vi "Q14070-Z040轴向间隙测试台.vi"() -> ()   [LabVIEW 2013]
uses:
  <vilib>/Utility/file.llb/Write To Spreadsheet File (DBL).vi
  PCI8622_32.dll
panel:
  in  "确定按钮 3":bool
  in  "确定按钮 2":bool
  in  "确定按钮":bool
  in  "密码":string
  out "生产":bool
  out "source":string caption="源"
  out "code":i32 caption="代码"
  out "阻挡 2":bool
  out "error out 5":errorcluster
  out "型号数量":dbl
  in  "循环次数":u16
  out "旋转左极限位(mm)":dbl=-40.0
  out "旋转右极限位(mm)":dbl=60.0
  out "输入轴快进位置(mm)":dbl=-40.0
  out "输入轴初始位置(mm)":dbl=60.0
  out "输入轴最终位置（mm)":dbl format="%#.3f"
  out "左右基准":dbl=-40.0
  in  "进给速度":dbl=10.0
  in  "旋转速度":dbl=10.0
  out "DeviceHandle":u32
  out "输入轴电机慢进位置3":dbl format="%#.3f"
  out "输入轴电机慢进位置2":dbl format="%#.3f"
  out "旋转轴伺服位置":dbl=10000.0 format="%#.2f"
  out "复位按钮":bool=TRUE
  out "报警工步号":dbl
  out "报警信息":string
  out "输入轴伺服位置":dbl=10000.0 format="%#.1f"
  out "力矩（nm)":dbl format="%#.2f"
  out "位移(mm)":dbl format="%#.3f"
  in  "员工权限":bool=TRUE
  out "测试操作状态":string
  in  "测试 工步号":dbl
  out "通讯状态":bool
  in  "停止":bool
  out "流水线操作状态":string
  in  "流水线工步号":dbl
  in  "联线按钮":bool
  in  "选项卡控件 2":enum32{"间隙曲线", "手动", "传感器校验", "参数查询"}(tab)
  out "10Nm间隙值(mm)":dbl format="%#.3f"
  out "-10Nm间隙值(mm)":dbl format="%#.3f"
  out "检测扭矩(NM)":dbl format="%#.1f"
  out "轴向间隙值(mm)":dbl format="%#.3f"
  out "上序合格":bool
  out "上序不合格":bool
  out "本序合格":bool
  out "间隙合格标准值(mm)":dbl=0.2 format="%#.3f"
  out "换向扭矩(NM)":dbl format="%#.1f"
  out "XY图":cluster{dbl[], dbl[]}[](graph)
  out "本序已做":bool
  in  "旋转伺服使能":bool
  in  "输入轴使能":bool
  out "放行":bool
  in  "阻挡":bool
  in  "扳手无效":bool
  out "流水线气缸下限":bool
  out "流水线气缸上限":bool
  out "下工位检测":bool
  out "本工位检测":bool
  out "上工位检测":bool
  in  "M顶升气缸上升":bool
  in  "M顶升气缸下降":bool
  in  "M本阻挡器":bool
  in  "M上阻挡器":bool
  in  "电机回零":bool
  in  "电机下降":bool
  in  "电机上升":bool
  in  "左旋":bool
  in  "右旋":bool
  in  "扭矩传感器零点偏移":dbl format="%#.2f"
  in  "扭矩传感器比例偏移":dbl=1.0 format="%#.2f"
  in  "位移传感器零点偏移":dbl format="%#.2f"
  in  "位移传感器比例偏移":dbl=1.0 format="%#.2f"
  in  "传感器参数保存":bool
  in  "参数保存":bool
  in  "参数查询":bool
  in  "参数列表":string[][](table)
  out "员工ID":string
  out "员工姓名":string
  in  "型号选择":u16(ring) items=["J728", "J706", "J709"]
  in  "参数加载":bool
  out "产品ID":string
  out "轴向间隙比例系数":dbl=1.0 format="%#_2f"
  out "error out 2":errorcluster
  out "输入轴电机快进速度":dbl format="%#.1f"
  out "输入轴电机慢进速度":dbl format="%#.3f"
  out "旋转电机速度":dbl=5.0 format="%#.3f"
  out "ADODB._Connection Out":refnum<k7>
  out "error out 3":errorcluster
  out "error out":errorcluster
  out "急停按钮":bool=TRUE
  out "芯片ID":string
  out "旋转轴AxisHandle OUT":u32
  out "FGCS":string="0"
  out "RFID读取完成":bool
  out "RFID读取触发":bool
  out "Z040 RFID":string="A001"
  out "KSJJ":string
  out "ReturnValue 3":u32
  out "ReturnValue":u32
  out "输入轴AxisHandle OUT":u32
  out "产品选型":dbl
  # "齿轮轴轴向间隙测试台"
  # "Q14070机械转向器装配线"
  # "Copying (C) 2015 湖北唯思凌科装备制造有限公司 版权所有"
  # "≤"
  # "传感器校验区"
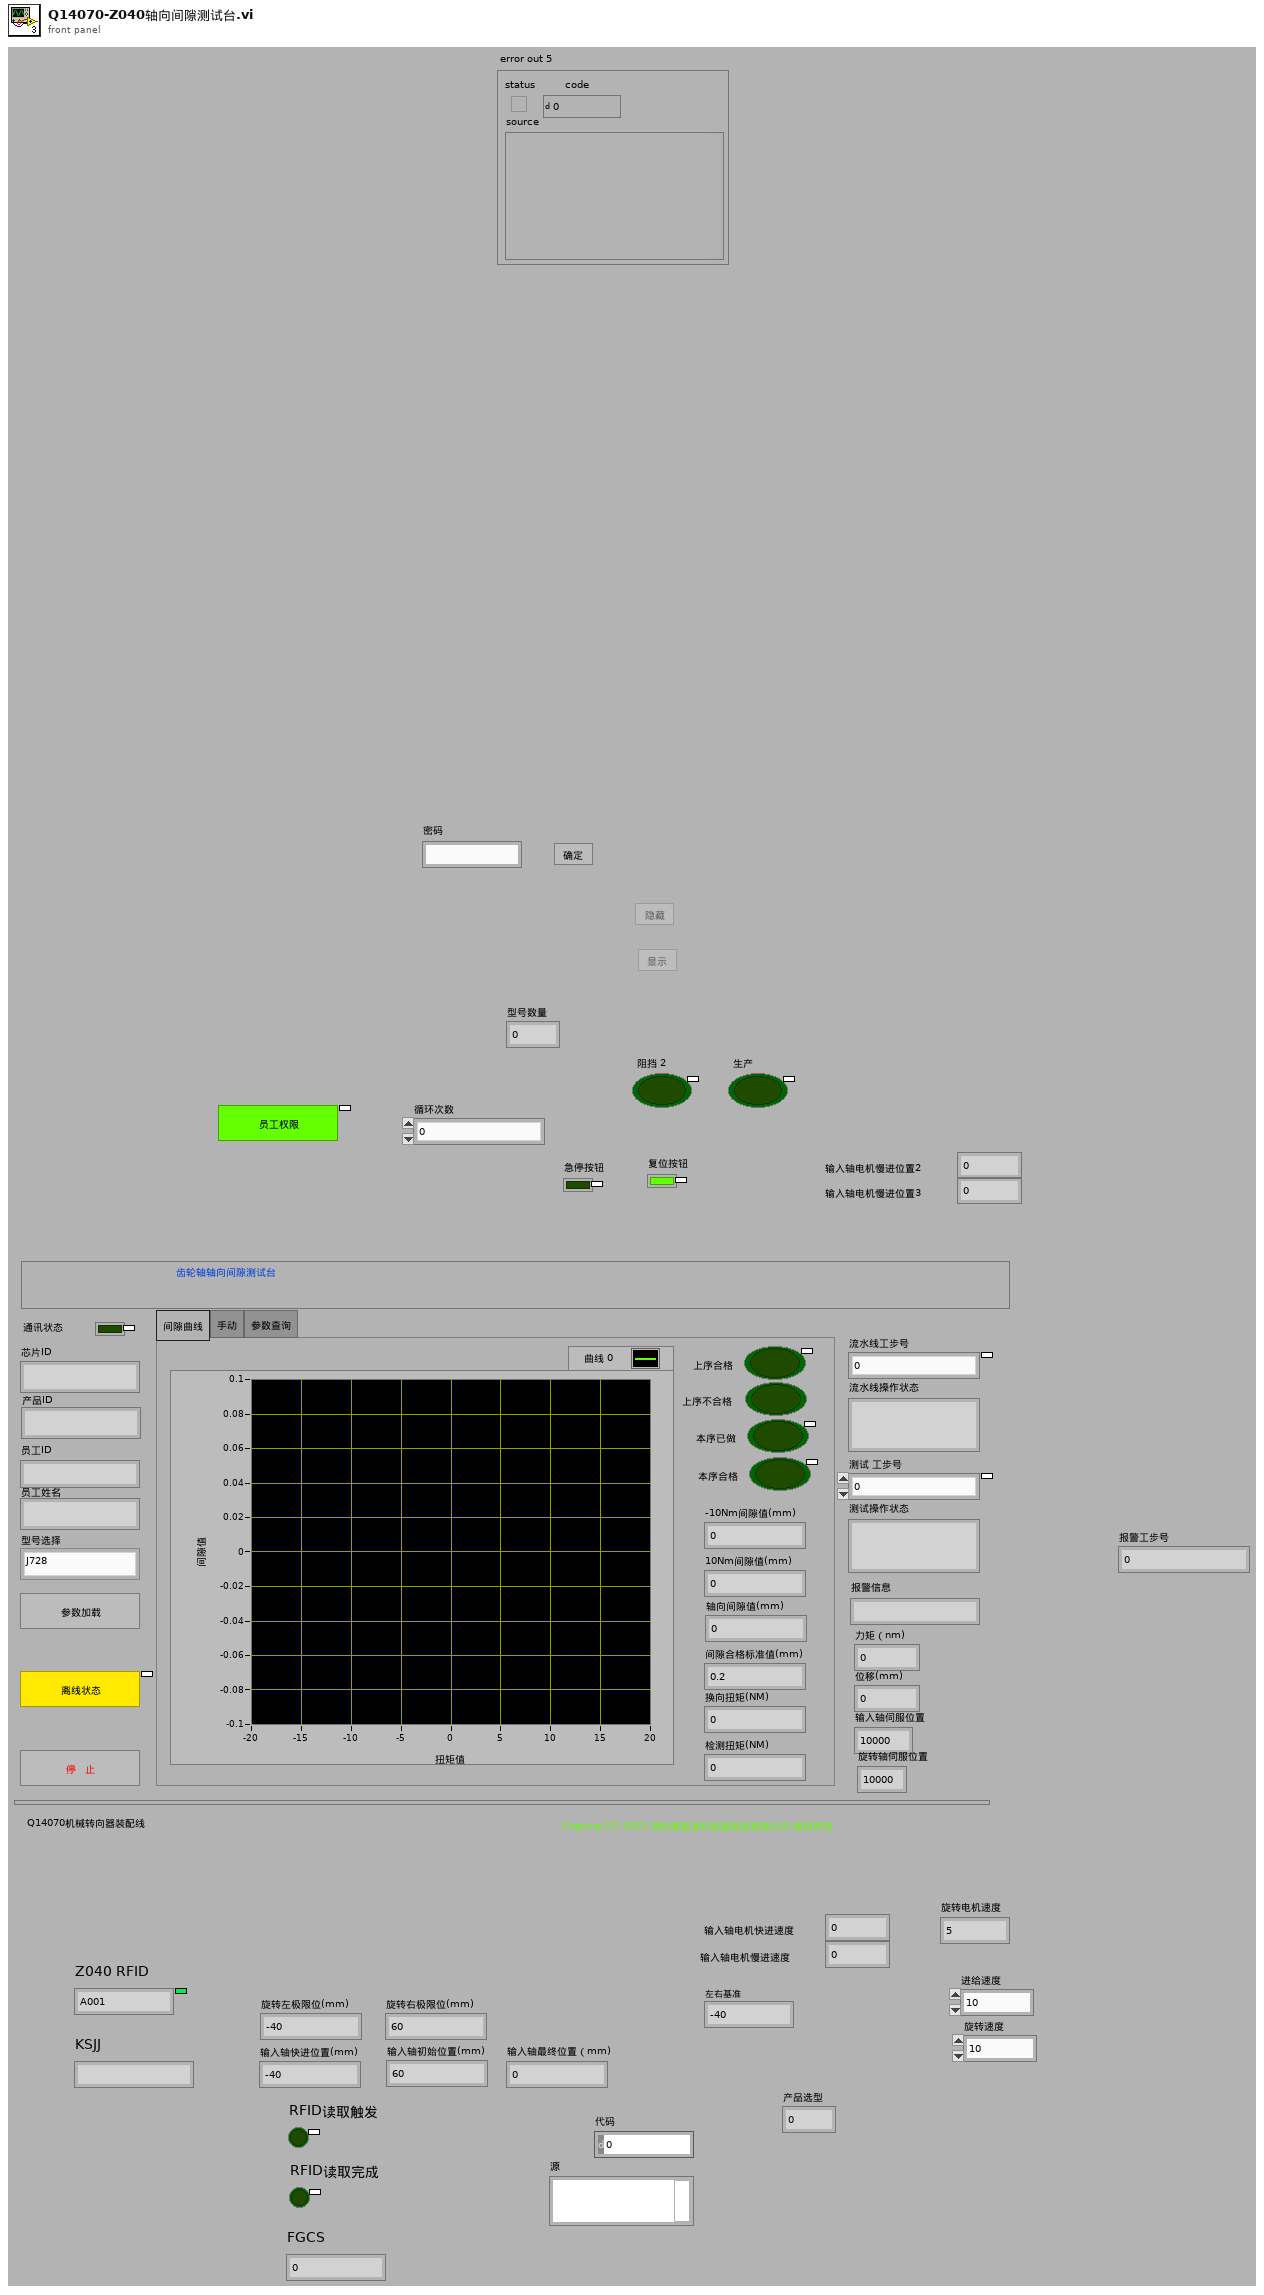
[diagram p1: front panel]
types:
  T1 = typedef "imagedata.ctl" = cluster{"image type":i32, "image depth":i32, "image":u8[], "mask":u8[], "colors":u32[], "Rectangle":cluster{"left":i16, "top":i16, "right":i16, "bottom":i16}}
  T2 = enum8{"Enabled", "Disabled", "Disabled and Grayed Out"}
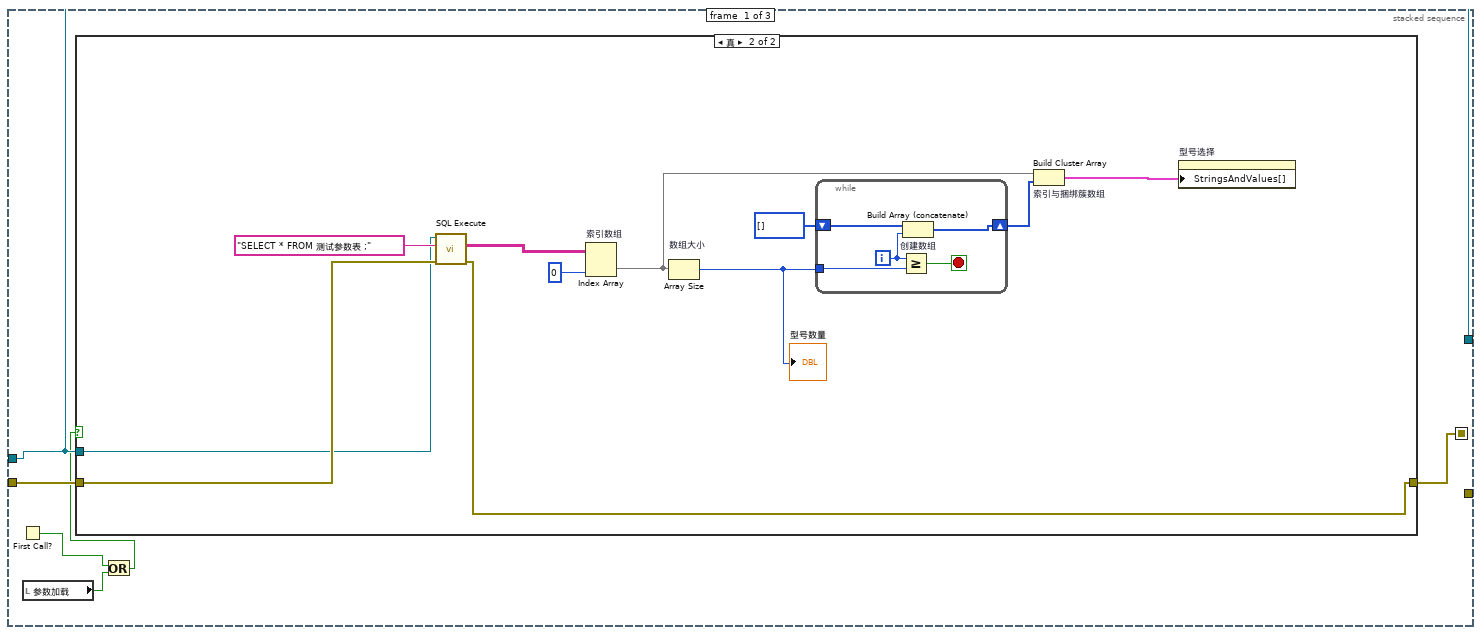
[diagram p3: hidden frame]
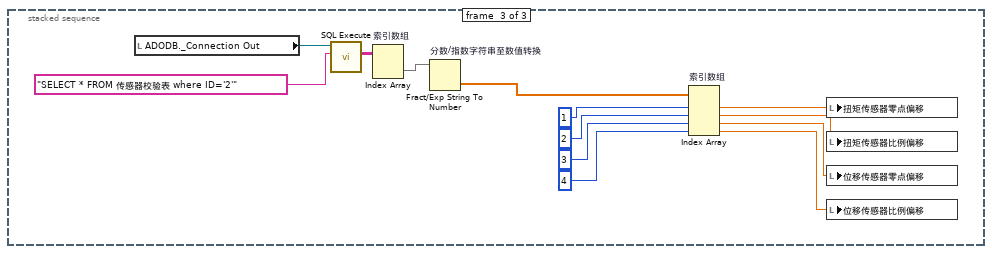
[diagram p5: hidden frame]
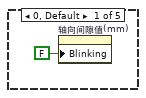
[diagram p6: hidden frame]
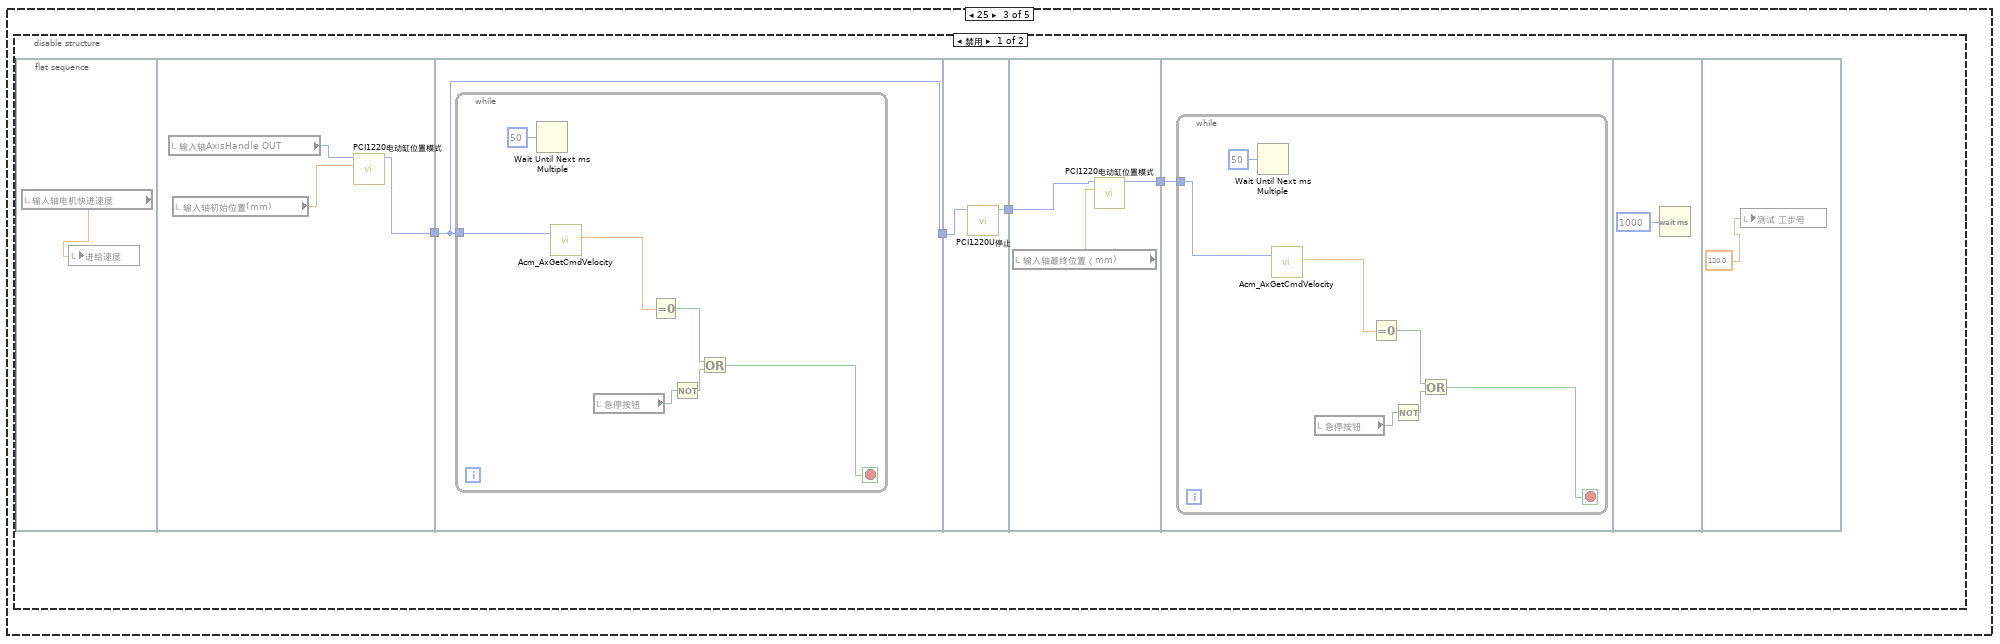
[diagram p8: hidden frame]
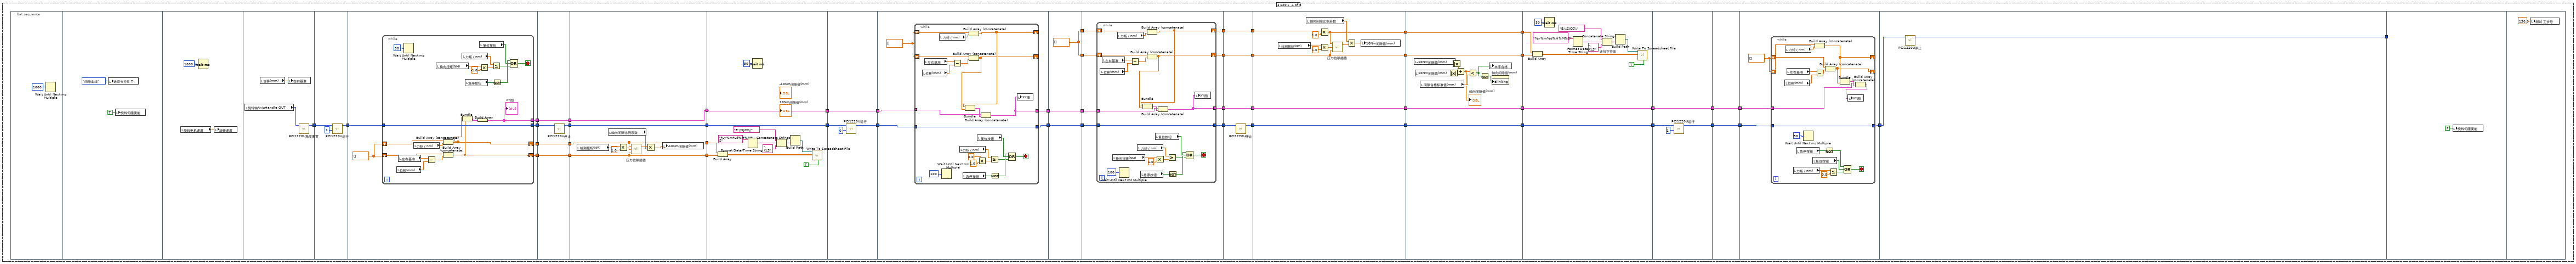
[diagram p10: hidden frame]
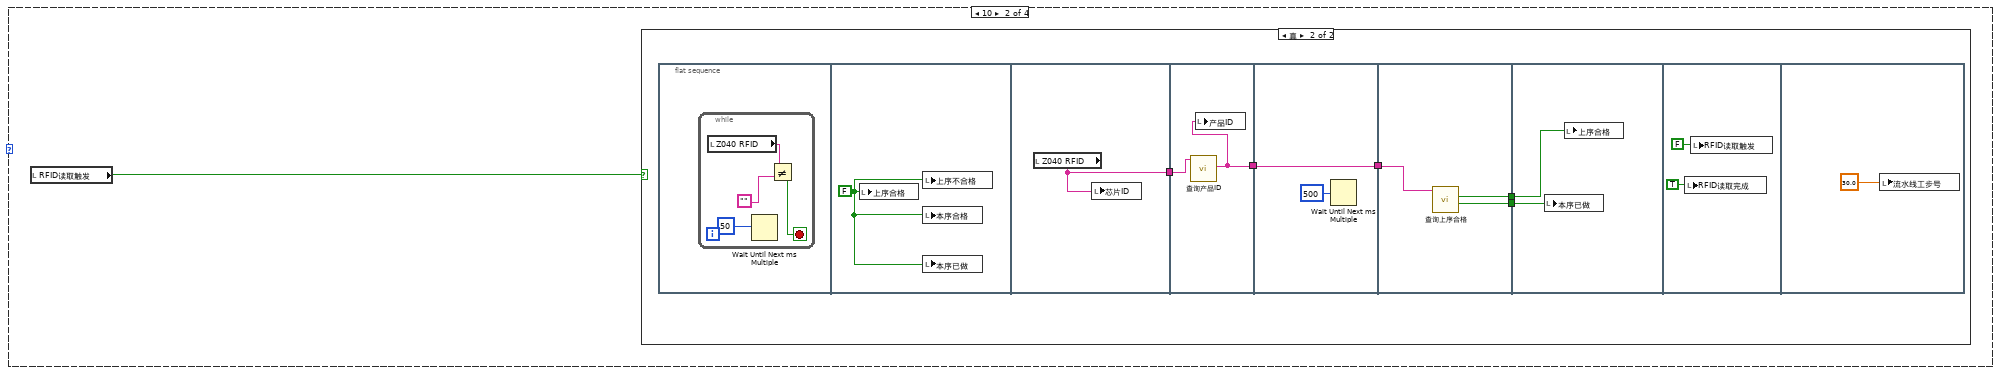
[diagram p12: hidden frame]
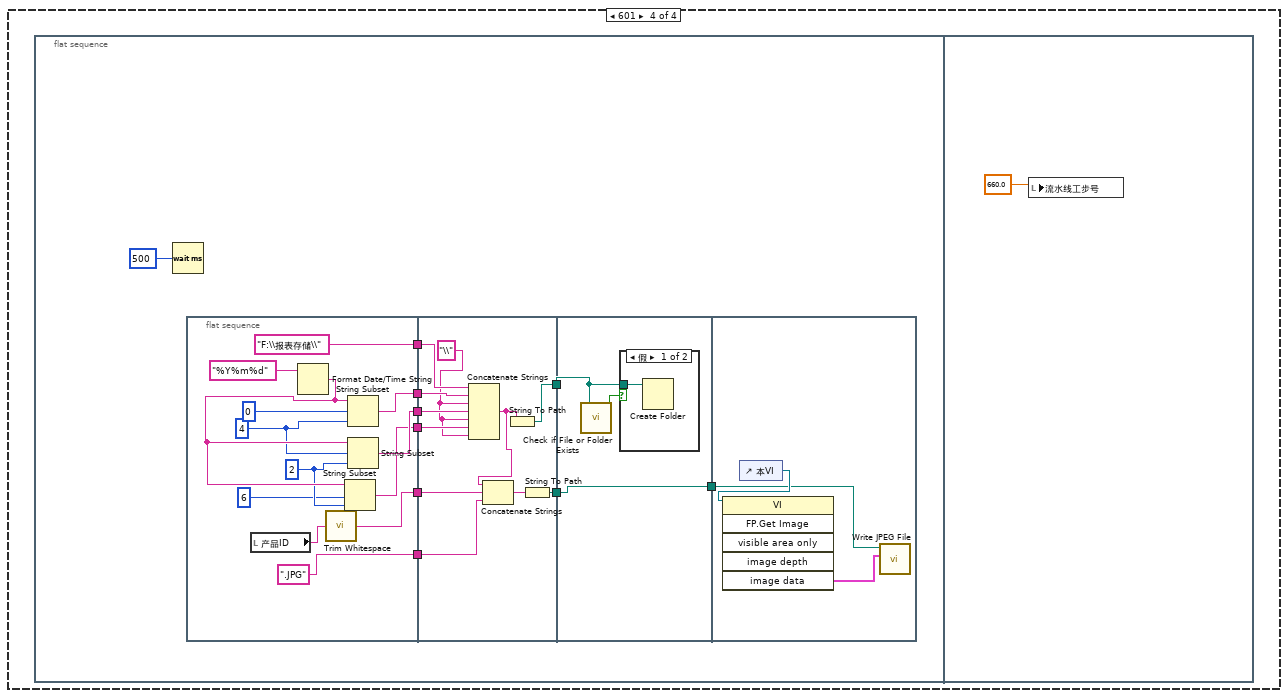
[diagram p15: hidden frame]
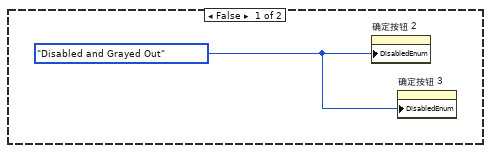
[diagram p17: hidden frame]
diagram:
  n1 = while {
    stop <- w10 stop-if-true
    n2 = local read "测试 工步号"() -> (w12:dbl)
    n3 = case shown="140" w12 {
      frame 0, Default {
        n4 = property on="轴向间隙值(mm)" class="DigNum (严格)"("Blinking"=FALSE ("闪烁")) -> ()  [unwired: 2 in, 2 out]
      }
      frame 20 {
        n5 = flat-sequence {
          tunnel: [w43] -> w14
          tunnel: w14 -> [w45]
          tunnel: [w45] -> w33
          tunnel: w33 -> [w47]
          tunnel: [w46] -> w35
          tunnel: w35 -> [w62]
          tunnel: [w64] -> w25
          tunnel: w25 -> [w67]
          tunnel: [w67] -> w24
          tunnel: w24 -> [w70]
          tunnel: [w70] -> w23
          tunnel: [w74] -> w30
          tunnel: w23 -> [w73]
          tunnel: [w71] -> w27
          tunnel: [w77] -> w32
          tunnel: w30 -> [w77]
          tunnel: [w78] -> w29
          tunnel: w27 -> [w78]
          tunnel: w32 -> [w81]
          tunnel: [w81] -> w31
          tunnel: w29 -> [w79]
          tunnel: [w79] -> w28
          tunnel: w31 -> [w85]
          tunnel: [w84] -> w34
          tunnel: w28 -> [w83]
          tunnel: [w82] -> w26
          tunnel: w34 -> [w104]
          tunnel: w26 -> [w101]
          tunnel: [w100] -> w22
          tunnel: w22 -> [w106]
          tunnel: [w106] -> w21
          tunnel: w21 -> [w107]
          tunnel: [w107] -> w20
          tunnel: w20 -> [w110]
          tunnel: [w110] -> w19
          tunnel: w19 -> [w112]
          tunnel: [w111] -> w15
          tunnel: w15 -> [w126]
          tunnel: [w125] -> w18
          tunnel: w18 -> [w128]
          tunnel: [w127] -> w17
          tunnel: w17 -> [w131]
          tunnel: [w131] -> w16
          tunnel: w16 -> [w132]
          frame #0 {
            w39 = 0.0
            n6 = local read "输入轴电机快进速度"() -> (w40:dbl)
            n7 = property on="轴向间隙值(mm)" class="DigNum (严格)"("Blinking"=FALSE ("闪烁")) -> ()  [unwired: 2 in, 2 out]
            n8 = Format Date/Time String(time format string (%c)="%Y%m%d%H%M" ("时间格式字符串(%c)")) -> (date/time string=w36:string)  [unwired: 2 in]
            n9 = local write "-10Nm间隙值(mm)"(w39) -> ()
            n10 = local write "10Nm间隙值(mm)"(w39) -> ()
            n11 = local write "轴向间隙值(mm)"(w39) -> ()
            n12 = local write "进给速度"(w40) -> ()
            n13 = local write "KSJJ"(w36) -> ()
          }
          frame #1 {
            n14 = local read "输入轴AxisHandle OUT"() -> (w41:u32)
            n15 = local read "输入轴快进位置(mm)"() -> (w42:dbl)
            n16 = call "PCI1220电动缸位置模式 .vi"("Distance"=w42, "AxisHandle IN"=w41) -> ("AxisHandle OUT"=w43:u32)  [unwired: 8 in, 1 out]
          }
          frame #2 {
            n17 = Wait (ms)(milliseconds to wait=u32 100 ("等待时间（毫秒）")) -> ()  [unwired: 1 out]
          }
          frame #3 {
            n18 = while {
              tunnel: w47 -> [w58]
              tunnel: [w59] -> w46
              stop <- w49 stop-if-true
              n19 = local read "力矩（nm)"() -> (w56:dbl)
              n20 = Wait Until Next ms Multiple(millisecond multiple=u32 50 ("毫秒倍数")) -> ()  [unwired: 1 out]
              n21 = Absolute Value(x=w56) -> (abs(x)=w55:dbl)
              n22 = call <userlib>:"Acm_AxGetCmdVelocity.vi"("AxisHandle"=w58) -> ("Velocity"=w60:dbl, "AxisHandle"=w59:u32)  [unwired: 1 in, 2 out]
              n23 = local read "急停按钮"() -> (w52:bool)
              n24 = Equal To 0?(x=w60) -> (x = 0?=w57:bool)
              n25 = local read "复位按钮"() -> (w48:bool)
              n26 = Greater Or Equal?(x=w55, y=15) -> (x >= y?=w53:bool)
              n27 = Or(x=w57, y=w53) -> (x .or. y?=w51:bool)
              n28 = Not(x=w52) -> (.not. x?=w50:bool)
              n29 = Compound Arithmetic op=OR(w48, w51, w50) -> (w49:bool)
            }
          }
          frame #4 {
            n30 = call "PCI1220U停止.vi"("AxisHandle IN"=w62) -> ()  [unwired: 9 in, 2 out]
          }
          frame #5 {
            n31 = local write "旋转伺服使能"(TRUE ("旋转伺服使能")) -> ()
          }
          frame #6 {
            n32 = local read "旋转轴AxisHandle OUT"() -> (w65:u32)
            n33 = call "PCI1220U角度置零.vi"("AxisHandle IN"=w65) -> ("AxisHandle OUT"=w64:u32)  [unwired: 10 in]
          }
          frame #7 {
            n34 = Wait (ms)(milliseconds to wait=u32 300 ("毫秒倍数")) -> ()  [unwired: 1 out]
          }
          frame #8 {
            n35 = local write "旋转速度"(2.0 ("旋转速度")) -> ()
            n36 = local read "输入轴电机慢进速度"() -> (w68:dbl)
            n37 = local write "进给速度"(w68) -> ()
          }
          frame #9 {
            n38 = local read "输入轴AxisHandle OUT"() -> (w76:u32)
            n39 = local read "输入轴最终位置（mm)"() -> (w75:dbl)
            n40 = call "PCI1220U旋转轴位置模式.vi"("Distance"=0.0, "AxisHandle IN"=w73) -> ("AxisHandle OUT"=w71:u32)  [unwired: 8 in, 1 out]
            n41 = call "PCI1220电动缸位置模式 .vi"("Distance"=w75, "AxisHandle IN"=w76) -> ("AxisHandle OUT"=w74:u32)  [unwired: 8 in, 1 out]
          }
          frame #10 {
          }
          frame #11 {
            n42 = Wait (ms)(milliseconds to wait=u32 100 ("等待时间（毫秒）")) -> ()  [unwired: 1 out]
          }
          frame #12 {
            n43 = while {
              tunnel: w85 -> [w99]
              tunnel: [w97] -> w84
              tunnel: w83 -> [w86]
              tunnel: [w86] -> w82
              stop <- w88 stop-if-true
              (unwired) u32 20 ("毫秒倍数")
              n44 = local read "力矩（nm)"() -> (w94:dbl)
              n45 = Absolute Value(x=w94) -> (abs(x)=w95:dbl)
              n46 = call <userlib>:"Acm_AxGetCmdVelocity.vi"("AxisHandle"=w99) -> ("Velocity"=w98:dbl, "AxisHandle"=w97:u32)  [unwired: 1 in, 2 out]
              n47 = local read "急停按钮"() -> (w92:bool)
              n48 = Equal To 0?(x=w98) -> (x = 0?=w87:bool)
              n49 = local read "复位按钮"() -> (w89:bool)
              n50 = Greater Or Equal?(x=w95, y=20) -> (x >= y?=w93:bool)
              n51 = Or(x=w87, y=w93) -> (x .or. y?=w91:bool)
              n52 = Not(x=w92) -> (.not. x?=w90:bool)
              n53 = Compound Arithmetic op=OR(w91, w90, w89) -> (w88:bool)
            }
          }
          frame #13 {
            n54 = call "PCI1220U停止.vi"("AxisHandle IN"=w104) -> ()  [unwired: 9 in, 2 out]
            n55 = local write "循环次数"(u16 0 ("循环次数")) -> ()
            n56 = Wait (ms)(milliseconds to wait=u32 200 ("毫秒计时值")) -> ()  [unwired: 1 out]
            n57 = call "PCI1220U停止.vi"("AxisHandle IN"=w101) -> ("AxisHandle OUT"=w100:u32)  [unwired: 9 in, 1 out]
          }
          frame #14 {
            n58 = Wait (ms)(milliseconds to wait=u32 200 ("毫秒计时值")) -> ()  [unwired: 1 out]
          }
          frame #15 {
            n59 = call "PCI1220U旋转轴位置模式.vi"("Distance"=-20.0, "AxisHandle IN"=w107) -> ()  [unwired: 8 in, 2 out]
          }
          frame #16 {
            n60 = Wait (ms)(milliseconds to wait=u32 100 ("毫秒计时值")) -> ()  [unwired: 1 out]
          }
          frame #17 {
            n61 = while {
              tunnel: w112 -> [w119]
              tunnel: [w115] -> w111
              stop <- w116 stop-if-true
              n62 = Wait Until Next ms Multiple(millisecond multiple=u32 20 ("毫秒倍数")) -> ()  [unwired: 1 out]
              n63 = local read "力矩（nm)"() -> (w122:dbl)
              n64 = local read "急停按钮"() -> (w114:bool)
              n65 = call <userlib>:"Acm_AxGetCmdVelocity.vi"("AxisHandle"=w119) -> ("Velocity"=w120:dbl, "AxisHandle"=w115:u32)  [unwired: 1 in, 2 out]
              n66 = Absolute Value(x=w122) -> (abs(x)=w121:dbl)
              n67 = Equal To 0?(x=w120) -> (x = 0?=w118:bool)
              n68 = Not(x=w114) -> (.not. x?=w113:bool)
              n69 = Greater Or Equal?(x=w121, y=u16 5) -> (x >= y?=w117:bool)
              n70 = Compound Arithmetic op=OR(w118, w117, w113) -> (w116:bool)
            }
          }
          frame #18 {
            n71 = call "PCI1220U停止.vi"("AxisHandle IN"=w126) -> ("AxisHandle OUT"=w125:u32)  [unwired: 9 in, 1 out]
          }
          frame #19 {
            n72 = call "PCI1220U旋转轴位置模式.vi"("Distance"=0.0, "AxisHandle IN"=w128) -> ("AxisHandle OUT"=w127:u32)  [unwired: 8 in, 1 out]
          }
          frame #20 {
            n73 = Wait (ms)(milliseconds to wait=u32 100 ("毫秒计时值")) -> ()  [unwired: 1 out]
          }
          frame #21 {
            n74 = while {
              tunnel: w132 -> [w135]
              tunnel: [w136] -> _
              stop <- w137 stop-if-true
              n75 = Wait Until Next ms Multiple(millisecond multiple=u32 20 ("毫秒倍数")) -> ()  [unwired: 1 out]
              n76 = local read "力矩（nm)"() -> (w142:dbl)
              n77 = local read "急停按钮"() -> (w134:bool)
              n78 = call <userlib>:"Acm_AxGetCmdVelocity.vi"("AxisHandle"=w135) -> ("Velocity"=w140:dbl, "AxisHandle"=w136:u32)  [unwired: 1 in, 2 out]
              n79 = Absolute Value(x=w142) -> (abs(x)=w141:dbl)
              n80 = Equal To 0?(x=w140) -> (x = 0?=w139:bool)
              n81 = Greater Or Equal?(x=w141, y=u16 5) -> (x >= y?=w138:bool)
              n82 = Not(x=w134) -> (.not. x?=w133:bool)
              n83 = Compound Arithmetic op=OR(w139, w138, w133) -> (w137:bool)
            }
          }
          frame #22 {
            n84 = local read "旋转轴AxisHandle OUT"() -> (w146:u32)
            n85 = local write "旋转伺服使能"(FALSE ("旋转伺服使能")) -> ()
            n86 = call "PCI1220U角度置零.vi"("AxisHandle IN"=w146) -> ()  [unwired: 10 in, 1 out]
          }
          frame #23 {
            n87 = Wait (ms)(milliseconds to wait=u32 1000 ("等待时间（毫秒）")) -> ()  [unwired: 1 out]
          }
          frame #24 {
            n88 = local write "测试 工步号"(120.0 ("流水线工步号")) -> ()
          }
        }
      }
      frame 25 {
        n89 = disable-structure shown="禁用" {
          frame Disabled {
            n90 = flat-sequence {
              tunnel: [w154] -> w152
              tunnel: w152 -> [w157]
              tunnel: [w157] -> w151
              tunnel: w151 -> [w166]
              tunnel: [w165] -> w150
              tunnel: w150 -> [w169]
              tunnel: [w167] -> w149
              tunnel: w149 -> [w170]
              frame #0 {
                n91 = local read "输入轴电机快进速度"() -> (w153:dbl)
                n92 = local write "进给速度"(w153) -> ()
              }
              frame #1 {
                n93 = local read "输入轴AxisHandle OUT"() -> (w156:u32)
                n94 = local read "输入轴初始位置(mm)"() -> (w155:dbl)
                n95 = call "PCI1220电动缸位置模式 .vi"("Distance"=w155, "AxisHandle IN"=w156) -> ("AxisHandle OUT"=w154:u32)  [unwired: 8 in, 1 out]
              }
              frame #2 {
                n96 = while {
                  tunnel: w157 -> [w160]
                  stop <- w163 stop-if-true
                  n97 = Wait Until Next ms Multiple(millisecond multiple=u32 50 ("毫秒倍数")) -> ()  [unwired: 1 out]
                  n98 = call <userlib>:"Acm_AxGetCmdVelocity.vi"("AxisHandle"=w160) -> ("Velocity"=w162:dbl)  [unwired: 1 in, 3 out]
                  n99 = local read "急停按钮"() -> (w164:bool)
                  n100 = Equal To 0?(x=w162) -> (x = 0?=w161:bool)
                  n101 = Not(x=w164) -> (.not. x?=w159:bool)
                  n102 = Or(x=w161, y=w159) -> (x .or. y?=w163:bool)
                }
              }
              frame #3 {
                n103 = call "PCI1220U停止.vi"("AxisHandle IN"=w166) -> ("AxisHandle OUT"=w165:u32)  [unwired: 9 in, 1 out]
              }
              frame #4 {
                n104 = local read "输入轴最终位置（mm)"() -> (w168:dbl)
                n105 = call "PCI1220电动缸位置模式 .vi"("Distance"=w168, "AxisHandle IN"=w169) -> ("AxisHandle OUT"=w167:u32)  [unwired: 8 in, 1 out]
              }
              frame #5 {
                n106 = while {
                  tunnel: w170 -> [w171]
                  stop <- w176 stop-if-true
                  n107 = Wait Until Next ms Multiple(millisecond multiple=u32 50 ("毫秒倍数")) -> ()  [unwired: 1 out]
                  n108 = call <userlib>:"Acm_AxGetCmdVelocity.vi"("AxisHandle"=w171) -> ("Velocity"=w175:dbl)  [unwired: 1 in, 3 out]
                  n109 = local read "急停按钮"() -> (w177:bool)
                  n110 = Equal To 0?(x=w175) -> (x = 0?=w174:bool)
                  n111 = Not(x=w177) -> (.not. x?=w173:bool)
                  n112 = Or(x=w174, y=w173) -> (x .or. y?=w176:bool)
                }
              }
              frame #6 {
                n113 = Wait (ms)(milliseconds to wait=u32 1000 ("等待时间（毫秒）")) -> ()  [unwired: 1 out]
              }
              frame #7 {
                n114 = local write "测试 工步号"(120.0 ("流水线工步号")) -> ()
              }
            }
          }
          frame Enabled {
          }
        }
      }
      frame 120 {
        n115 = flat-sequence {
          tunnel: [w235] -> w203
          tunnel: w203 -> [w237]
          tunnel: [w236] -> w211
          tunnel: w211 -> [w244]
          tunnel: [w243] -> w227
          tunnel: [w242] -> w226
          tunnel: [w241] -> w217
          tunnel: [w240] -> w200
          tunnel: w227 -> [w270]
          tunnel: w226 -> [w269]
          tunnel: [w269] -> w225
          tunnel: [w268] -> w224
          tunnel: [w267] -> w223
          tunnel: w217 -> [w268]
          tunnel: w200 -> [w266]
          tunnel: [w266] -> w199
          tunnel: w225 -> [w273]
          tunnel: w224 -> [w274]
          tunnel: w223 -> [w280]
          tunnel: [w280] -> w207
          tunnel: [w274] -> w205
          tunnel: [w273] -> w204
          tunnel: w199 -> [w272]
          tunnel: [w272] -> w198
          tunnel: w207 -> [w293]
          tunnel: [w293] -> w206
          tunnel: w205 -> [w285]
          tunnel: w204 -> [w284]
          tunnel: [w282] -> w202
          tunnel: w198 -> [w282]
          tunnel: w206 -> [w296]
          tunnel: [w295] -> w197
          tunnel: w202 -> [w294]
          tunnel: [w294] -> w195
          tunnel: w197 -> [w302]
          tunnel: [w299] -> w196
          tunnel: w195 -> [w301]
          tunnel: [w300] -> w194
          tunnel: [w327] -> w219
          tunnel: [w325] -> w218
          tunnel: [w325] -> w212
          tunnel: w196 -> [w327]
          tunnel: [w326] -> w201
          tunnel: w194 -> [w326]
          tunnel: w219 -> [w335]
          tunnel: w218 -> [w333]
          tunnel: [w334] -> w222
          tunnel: [w331] -> w221
          tunnel: [w330] -> w220
          tunnel: w212 -> [w332]
          tunnel: w201 -> [w329]
          tunnel: [w328] -> w193
          tunnel: w222 -> [w362]
          tunnel: w221 -> [w361]
          tunnel: [w361] -> w210
          tunnel: w220 -> [w360]
          tunnel: [w360] -> w209
          tunnel: [w359] -> w208
          tunnel: w193 -> [w358]
          tunnel: [w358] -> w192
          tunnel: w210 -> [w368]
          tunnel: w209 -> [w370]
          tunnel: [w373] -> w188
          tunnel: w208 -> [w373]
          tunnel: [w369] -> w186
          tunnel: [w368] -> w184
          tunnel: w192 -> [w364]
          tunnel: [w364] -> w182
          tunnel: w188 -> [w386]
          tunnel: [w386] -> w187
          tunnel: w186 -> [w385]
          tunnel: [w385] -> w185
          tunnel: w184 -> [w384]
          tunnel: [w384] -> w183
          tunnel: w182 -> [w383]
          tunnel: [w383] -> w181
          tunnel: [w399] -> w216
          tunnel: w187 -> [w399]
          tunnel: w185 -> [w392]
          tunnel: w183 -> [w391]
          tunnel: w181 -> [w387]
          tunnel: [w387] -> w191
          tunnel: w216 -> [w402]
          tunnel: [w401] -> w214
          tunnel: w191 -> [w400]
          tunnel: [w400] -> w190
          tunnel: [w405] -> w215
          tunnel: w214 -> [w405]
          tunnel: w190 -> [w404]
          tunnel: [w404] -> w189
          tunnel: w215 -> [w409]
          tunnel: [w408] -> w213
          tunnel: w189 -> [w406]
          tunnel: w213 -> [w431]
          tunnel: [w430] -> w180
          tunnel: w180 -> [_]
          frame #0 {
            n116 = Wait Until Next ms Multiple(millisecond multiple=u32 1000 ("毫秒倍数")) -> ()  [unwired: 1 out]
          }
          frame #1 {
            n117 = local write "选项卡控件 2"(enum32{"间隙曲线", "手动", "传感器校验", "参数查询"}."间隙曲线" ("选项卡控件 2")) -> ()
            n118 = local write "旋转伺服使能"(TRUE ("旋转伺服使能")) -> ()
          }
          frame #2 {
            n119 = local read "旋转电机速度"() -> (w232:dbl)
            n120 = Wait (ms)(milliseconds to wait=u32 1000 ("毫秒倍数")) -> ()  [unwired: 1 out]
            n121 = local write "旋转速度"(w232) -> ()
          }
          frame #3 {
            n122 = local read "旋转轴AxisHandle OUT"() -> (w233:u32)
            n123 = local read "位移(mm)"() -> (w234:dbl)
            n124 = local write "左右基准"(w234) -> ()
            n125 = call "PCI1220U角度置零.vi"("AxisHandle IN"=w233) -> ("AxisHandle OUT"=w235:u32)  [unwired: 10 in]
          }
          frame #4 {
            n126 = call "PCI1220U运行.vi"("方向"=u16 1, "AxisHandle IN"=w237) -> ("AxisHandle OUT"=w236:u32)  [unwired: 9 in]
          }
          frame #5 {
            w239 = dbl[] [] ("添加的数组")
            n127 = while {
              tunnel: w244 -> [w258]
              tunnel: [w258] -> w243
              shift-right: [w247] -> w241
              shift-left: w239 -> [w248]
              shift-right: [w246] -> w242
              shift-left: w239 -> [w252]
              tunnel: [w245] -> w240
              stop <- w253 stop-if-true
              n128 = local read "位移(mm)"() -> (w251:dbl)
              n129 = local read "左右基准"() -> (w250:dbl)
              n130 = Wait Until Next ms Multiple(millisecond multiple=u32 50 ("毫秒倍数")) -> ()  [unwired: 1 out]
              n131 = local read "力矩（nm)"() -> (w265:dbl)
              n132 = Subtract(x=w250, y=w251) -> (x-y=w263:dbl)
              n133 = local read "换向扭矩(NM)"() -> (w262:dbl)
              n134 = Build Array (concatenate)(w248, w265) -> (w247:dbl[])
              n135 = Build Array (concatenate)(w252, w263) -> (w246:dbl[])
              n136 = local read "力矩（nm)"() -> (w260:dbl)
              n137 = Bundle(w247, w246) -> (w249:cluster{dbl[], dbl[]})  [unwired: 1 in]
              n138 = local read "急停按钮"() -> (w257:bool)
              n139 = Build Array(w249) -> (w245:cluster{dbl[], dbl[]}[])
              "XY图" <- w245
              n140 = local read "复位按钮"() -> (w255:bool)
              n141 = Multiply(x=w262, y=-1.0) -> (x*y=w259:dbl)
              n142 = Less Or Equal?(x=w260, y=w259) -> (x <= y?=w254:bool)
              n143 = Not(x=w257) -> (.not. x?=w256:bool)
              n144 = Compound Arithmetic op=OR(w256, w255, w254) -> (w253:bool)
            }
          }
          frame #6 {
            n145 = call "PCI1220U停止.vi"("AxisHandle IN"=w270) -> ("AxisHandle OUT"=w267:u32)  [unwired: 9 in, 1 out]
          }
          frame #7 {
            n146 = local read "检测扭矩(NM)"() -> (w275:dbl)
            n147 = local read "轴向间隙比例系数"() -> (w278:dbl)
            n148 = Multiply(x=w275, y=1.0) -> (x*y=w277:dbl)
            n149 = call "压力位移插值.vi"("压力数组"=w273, "监控点位移"=w277, "位移数组"=w274) -> ("监控点压力"=w279:dbl)  [unwired: 2 in]
            n150 = Multiply(x=w278, y=w279) -> (x*y=w271:dbl)
            n151 = local write "-10Nm间隙值(mm)"(w271) -> ()
          }
          frame #8 {
            n152 = Build Array(w285, w284) -> (w283:dbl[][])
            n153 = Format Date/Time String(time format string (%c)="%y%m%d%H%M%S" ("时间格式字符串(%c)")) -> (date/time string=w292:string)  [unwired: 2 in]
            n154 = Wait (ms)(milliseconds to wait=u32 50 ("等待时间（毫秒）")) -> ()  [unwired: 1 out]
            n155 = Concatenate Strings("E:\\SJCC\\" ("时间格式字符串(%c)"), w292, ".XLS") -> (w287:string)
            n156 = Build Path(name or relative path=w287) -> (appended path=w288:path)  [unwired: 1 in]
            n157 = call-poly <vilib>:"Write To Spreadsheet File.vi"("transpose? (no:F)"=TRUE, "2D data"=w283, "file path (dialog if empty)"=w288) -> ()  [unwired: 5 in, 1 out]
          }
          frame #9 {
            n158 = call "PCI1220U运行.vi"("方向"=u16 0, "AxisHandle IN"=w296) -> ("AxisHandle OUT"=w295:u32)  [unwired: 9 in]
          }
          frame #10 {
            w298 = dbl[] [] ("添加的数组")
            n159 = while {
              tunnel: w302 -> [w319]
              tunnel: [w319] -> w299
              shift-right: [w308] -> _
              shift-left: w298 -> [w313]
              shift-right: [w307] -> _
              shift-left: w298 -> [w312]
              tunnel: w301 -> [w304]
              tunnel: [w306] -> w300
              stop <- w314 stop-if-true
              n160 = local read "位移(mm)"() -> (w310:dbl)
              n161 = local read "左右基准"() -> (w309:dbl)
              n162 = local read "力矩（nm)"() -> (w324:dbl)
              n163 = Wait Until Next ms Multiple(millisecond multiple=u32 100 ("毫秒倍数")) -> ()  [unwired: 1 out]
              n164 = Subtract(x=w309, y=w310) -> (x-y=w311:dbl)
              n165 = local read "力矩（nm)"() -> (w322:dbl)
              n166 = local read "急停按钮"() -> (w316:bool)
              n167 = Build Array (concatenate)(w313, w324) -> (w308:dbl[])
              n168 = Build Array (concatenate)(w312, w311) -> (w307:dbl[])
              n169 = Bundle(w308, w307) -> (w303:cluster{dbl[], dbl[]})  [unwired: 1 in]
              n170 = local read "复位按钮"() -> (w318:bool)
              n171 = Multiply(x=0.0, y=1.0) -> (x*y=w320:dbl)
              n172 = Build Array (concatenate)(w304, w303) -> (w306:cluster{dbl[], dbl[]}[])
              n173 = Greater Or Equal?(x=w322, y=w320) -> (x >= y?=w315:bool)
              n174 = Not(x=w316) -> (.not. x?=w317:bool)
              n175 = Compound Arithmetic op=OR(w317, w318, w315) -> (w314:bool)
              n176 = local write "XY图"(w306) -> ()
            }
          }
          frame #11 {
            w325 = dbl[] [] ("添加的数组")
          }
          frame #12 {
            n177 = while {
              tunnel: w335 -> [w351]
              tunnel: [w351] -> w334
              shift-right: [w340] -> w330
              shift-left: w333 -> [w345]
              shift-right: [w339] -> w331
              shift-left: w332 -> [w344]
              tunnel: w329 -> [w336]
              tunnel: [w338] -> w328
              stop <- w346 stop-if-true
              n178 = local read "位移(mm)"() -> (w342:dbl)
              n179 = local read "左右基准"() -> (w341:dbl)
              n180 = local read "换向扭矩(NM)"() -> (w354:dbl)
              n181 = local read "力矩（nm)"() -> (w357:dbl)
              n182 = Wait Until Next ms Multiple(millisecond multiple=u32 100 ("毫秒倍数")) -> ()  [unwired: 1 out]
              n183 = Subtract(x=w341, y=w342) -> (x-y=w343:dbl)
              n184 = local read "力矩（nm)"() -> (w355:dbl)
              n185 = local read "急停按钮"() -> (w348:bool)
              n186 = Build Array (concatenate)(w345, w357) -> (w340:dbl[])
              n187 = Build Array (concatenate)(w344, w343) -> (w339:dbl[])
              n188 = Bundle(w340, w339) -> (w337:cluster{dbl[], dbl[]})  [unwired: 1 in]
              n189 = local read "复位按钮"() -> (w350:bool)
              n190 = Multiply(x=w354, y=1.0) -> (x*y=w352:dbl)
              n191 = Build Array (concatenate)(w336, w337) -> (w338:cluster{dbl[], dbl[]}[])
              n192 = Greater Or Equal?(x=w355, y=w352) -> (x >= y?=w347:bool)
              n193 = Not(x=w348) -> (.not. x?=w349:bool)
              n194 = Compound Arithmetic op=OR(w349, w350, w347) -> (w346:bool)
              n195 = local write "XY图"(w338) -> ()
            }
          }
          frame #13 {
            n196 = call "PCI1220U停止.vi"("AxisHandle IN"=w362) -> ("AxisHandle OUT"=w359:u32)  [unwired: 9 in, 1 out]
          }
          frame #14 {
            n197 = local read "检测扭矩(NM)"() -> (w367:dbl)
            n198 = local read "轴向间隙比例系数"() -> (w374:dbl)
            n199 = Multiply(x=w370, y=1.0) -> (x*y=w369:dbl[])
            n200 = Multiply(x=w367, y=1.0) -> (x*y=w366:dbl)
            n201 = call "压力位移插值.vi"("压力数组"=w368, "监控点位移"=w366, "位移数组"=w369) -> ("监控点压力"=w372:dbl)  [unwired: 2 in]
            n202 = Multiply(x=w374, y=w372) -> (x*y=w363:dbl)
            n203 = local write "10Nm间隙值(mm)"(w363) -> ()
          }
          frame #15 {
            n204 = local read "-10Nm间隙值(mm)"() -> (w381:dbl)
            n205 = local read "10Nm间隙值(mm)"() -> (w382:dbl)
            n206 = local read "间隙合格标准值(mm)"() -> (w380:dbl)
            n207 = Absolute Value(x=w382) -> (abs(x)=w377:dbl)
            n208 = Absolute Value(x=w381) -> (abs(x)=w378:dbl)
            n209 = Add(x=w378, y=w377) -> (x+y=w379:dbl)
            "轴向间隙值(mm)" <- w379
            n210 = Less?(x=w379, y=w380) -> (x < y?=w376:bool)
            n211 = Not(x=w376) -> (.not. x?=w375:bool)
            n212 = local write "本序合格"(w376) -> ()
            n213 = property on="轴向间隙值(mm)" class="DigNum (严格)"("Blinking"=w375) -> ()  [unwired: 2 in, 2 out]
          }
          frame #16 {
            n214 = Build Array(w392, w391) -> (w393:dbl[][])
            n215 = Wait (ms)(milliseconds to wait=u32 50 ("等待时间（毫秒）")) -> ()  [unwired: 1 out]
            n216 = Format Date/Time String(time format string (%c)="%y%m%d%H%M%S" ("时间格式字符串(%c)")) -> (date/time string=w389:string)  [unwired: 2 in]
            n217 = Concatenate Strings "连接字符串"("E:\\SJCC\\" ("时间格式字符串(%c)"), w389, ".XLS") -> (w397:string)
            n218 = Build Path(name or relative path=w397) -> (appended path=w396:path)  [unwired: 1 in]
            n219 = call-poly <vilib>:"Write To Spreadsheet File.vi"("transpose? (no:F)"=TRUE, "2D data"=w393, "file path (dialog if empty)"=w396) -> ()  [unwired: 5 in, 1 out]
          }
          frame #17 {
            n220 = call "PCI1220U运行.vi"("方向"=u16 1, "AxisHandle IN"=w402) -> ("AxisHandle OUT"=w401:u32)  [unwired: 9 in]
          }
          frame #18 {
          }
          frame #19 {
            w407 = dbl[] [] ("添加的数组")
            n221 = while {
              tunnel: w409 -> [w427]
              tunnel: [w427] -> w408
              shift-right: [w411] -> _
              shift-left: w407 -> [w416]
              shift-right: [w410] -> _
              shift-left: w407 -> [w415]
              tunnel: w406 -> [w412]
              stop <- w422 stop-if-true
              n222 = local read "位移(mm)"() -> (w419:dbl)
              n223 = local read "力矩（nm)"() -> (w417:dbl)
              n224 = local read "左右基准"() -> (w420:dbl)
              n225 = local read "力矩（nm)"() -> (w428:dbl)
              n226 = local read "急停按钮"() -> (w424:bool)
              n227 = Wait Until Next ms Multiple(millisecond multiple=u32 50 ("毫秒倍数")) -> ()  [unwired: 1 out]
              n228 = local read "复位按钮"() -> (w426:bool)
              n229 = Build Array (concatenate)(w416, w417) -> (w411:dbl[])
              n230 = Subtract(x=w420, y=w419) -> (x-y=w418:dbl)
              n231 = Not(x=w424) -> (.not. x?=w425:bool)
              n232 = Build Array (concatenate)(w415, w418) -> (w410:dbl[])
              n233 = Less Or Equal?(x=w428, y=0.0) -> (x <= y?=w423:bool)
              n234 = Bundle(w411, w410) -> (w413:cluster{dbl[], dbl[]})  [unwired: 1 in]
              n235 = Compound Arithmetic op=OR(w425, w426, w423) -> (w422:bool)
              n236 = Build Array (concatenate)(w412, w413) -> (w414:cluster{dbl[], dbl[]}[])
              n237 = local write "XY图"(w414) -> ()
            }
          }
          frame #20 {
            n238 = call "PCI1220U停止.vi"("AxisHandle IN"=w431) -> ("AxisHandle OUT"=w430:u32)  [unwired: 9 in, 1 out]
          }
          frame #21 {
            n239 = local write "旋转伺服使能"(FALSE ("旋转伺服使能")) -> ()
          }
          frame #22 {
            n240 = local write "测试 工步号"(130.0 ("测试 工步号")) -> ()
          }
        }
      }
      frame 140 {
        n241 = flat-sequence {
          tunnel: [w438] -> w434
          tunnel: [w440] -> w435
          tunnel: w434 -> [w440]
          tunnel: w435 -> [w442]
          frame #0 {
            n242 = local read "输入轴电机快进速度"() -> (w436:dbl)
            n243 = local write "进给速度"(w436) -> ()
          }
          frame #1 {
            n244 = local read "输入轴AxisHandle OUT"() -> (w439:u32)
            n245 = local read "输入轴初始位置(mm)"() -> (w437:dbl)
            n246 = call "PCI1220电动缸位置模式 .vi"("Distance"=w437, "AxisHandle IN"=w439) -> ("AxisHandle OUT"=w438:u32)  [unwired: 8 in, 1 out]
          }
          frame #2 {
            n247 = Wait (ms)(milliseconds to wait=u32 50 ("毫秒倍数")) -> ()  [unwired: 1 out]
          }
          frame #3 {
            n248 = while {
              tunnel: w442 -> [w449]
              stop <- w443 stop-if-true
              n249 = call <userlib>:"Acm_AxGetCmdVelocity.vi"("AxisHandle"=w449) -> ("Velocity"=w448:dbl)  [unwired: 1 in, 3 out]
              n250 = local read "急停按钮"() -> (w447:bool)
              n251 = Wait Until Next ms Multiple(millisecond multiple=u32 50 ("毫秒倍数")) -> ()  [unwired: 1 out]
              n252 = local read "复位按钮"() -> (w444:bool)
              n253 = Equal To 0?(x=w448) -> (x = 0?=w446:bool)
              n254 = Not(x=w447) -> (.not. x?=w445:bool)
              n255 = Compound Arithmetic op=OR(w446, w445, w444) -> (w443:bool)
            }
          }
          frame #4 {
            n256 = Wait (ms)(milliseconds to wait=u32 50 ("毫秒倍数")) -> ()  [unwired: 1 out]
          }
          frame #5 {
            n257 = local write "测试 工步号"(990.0 ("测试 工步号")) -> ()
          }
        }
      }
    }
    n258 = Wait Until Next ms Multiple(millisecond multiple=u32 50 ("毫秒倍数")) -> ()  [unwired: 1 out]
    n259 = local read "停止"() -> (w10:bool)
  }
  n260 = while {
    stop <- w455 stop-if-true
    n261 = local read "流水线工步号"() -> (w453:dbl)
    n262 = case shown="600" w453 {
      frame 0, Default {
      }
      frame 10 {
        n263 = local read "RFID读取触发"() -> (w456:bool)
        n264 = case shown="真" w456 {
          frame False {
          }
          frame True {
            n265 = flat-sequence {
              tunnel: [w467] -> w461
              tunnel: w461 -> [w469]
              tunnel: [w468] -> w458
              tunnel: w458 -> [w471]
              tunnel: [w471] -> w457
              tunnel: w457 -> [w474]
              tunnel: [w473] -> w460
              tunnel: [w472] -> w459
              tunnel: w460 -> [w476]
              tunnel: w459 -> [w475]
              frame #0 {
                n266 = while {
                  stop <- w463 stop-if-true
                  n267 = local read "Z040 RFID"() -> (w465:string)
                  n268 = Wait Until Next ms Multiple(millisecond multiple=u32 50 ("毫秒计时值")) -> ()  [unwired: 1 out]
                  n269 = Not Equal?(x=w465, y="") -> (x != y?=w463:bool)
                }
              }
              frame #1 {
                w466 = FALSE ("上序合格")
                n270 = local write "上序合格"(w466) -> ()
                n271 = local write "上序不合格"(w466) -> ()
                n272 = local write "本序合格"(w466) -> ()
                n273 = local write "本序已做"(w466) -> ()
              }
              frame #2 {
                n274 = local read "Z040 RFID"() -> (w467:string)
                n275 = local write "芯片ID"(w467) -> ()
              }
              frame #3 {
                n276 = call "查询产品ID.vi"("芯片编码"=w469) -> ("产品ID"=w468:string)  [unwired: 8 in, 2 out]
                n277 = local write "产品ID"(w468) -> ()
              }
              frame #4 {
                n278 = Wait Until Next ms Multiple(millisecond multiple=u32 500 ("毫秒倍数")) -> ()  [unwired: 1 out]
              }
              frame #5 {
                n279 = call "查询上序合格.vi"("产品ID"=w474) -> ("本序已做"=w472:bool, "上序合格"=w473:bool)  [unwired: 8 in, 1 out]
              }
              frame #6 {
                n280 = local write "本序已做"(w475) -> ()
                n281 = local write "上序合格"(w476) -> ()
              }
              frame #7 {
                n282 = local write "RFID读取完成"(TRUE ("RFID读取完成")) -> ()
                n283 = local write "RFID读取触发"(FALSE ("RFID读取触发")) -> ()
              }
              frame #8 {
                n284 = local write "流水线工步号"(30.0 ("工步号")) -> ()
              }
            }
          }
        }
      }
      frame 600 {
        n285 = flat-sequence {
          tunnel: [w488] -> w480
          tunnel: w480 -> [w505]
          frame #0 {
            n286 = local read "本序合格"() -> (w491:bool)
            n287 = local read "轴向间隙值(mm)"() -> (w489:dbl)
            n288 = local read "KSJJ"() -> (w490:string)
            n289 = local read "产品ID"() -> (w487:string)
            n290 = local read "FGCS"() -> (w481:string)
            n291 = local read "员工ID"() -> (w492:string)
            n292 = Boolean To (0,1)(Boolean=w491) -> (0, 1=w494:i16)
            n293 = Number To Decimal String(number=w494, width (-)=i16 1 ("宽度(-)")) -> (decimal integer string=w485:string)
            n294 = Number To Fractional String(number=w489, precision (6)=i16 3 ("精度(6)")) -> (F-format string=w483:string)  [unwired: 2 in]
            n295 = Build Array(w487, w492, "1" ("元素"), w485, w490, w481, "Q14070-Z040", w483) -> (w488:string[])
          }
          frame #1 {
            n296 = call "数据库更新.vi"("设备号"="04", "数据"=w505) -> ()  [unwired: 13 in, 1 out]
            n297 = Wait (ms)(milliseconds to wait=u32 500 ("等待时间（毫秒）")) -> ()  [unwired: 1 out]
            n298 = flat-sequence {
              tunnel: ["F:\\报表存储\\"] -> w503
              tunnel: [w511] -> w502
              tunnel: [w510] -> w501
              tunnel: [w509] -> w500
              tunnel: [w508] -> w499
              tunnel: [".JPG"] -> w498
              tunnel: w503 -> [w529]
              tunnel: w502 -> [w528]
              tunnel: w501 -> [w527]
              tunnel: w500 -> [w526]
              tunnel: [w524] -> w497
              tunnel: w499 -> [w522]
              tunnel: w498 -> [w521]
              tunnel: [w519] -> w496
              tunnel: w497 -> [w531]
              tunnel: w496 -> [w530]
              tunnel: [w530] -> w495
              tunnel: w495 -> [w535]
              frame #0 {
                w514 = 2 ("长度（剩余）")
                w515 = 4 ("长度（剩余）")
                n299 = local read "产品ID"() -> (w508:string)
                n300 = Format Date/Time String(time format string (%c)="%Y%m%d") -> (date/time string=w516:string)  [unwired: 2 in]
                n301 = String Subset(string=w516, offset (0)=6 ("长度（剩余）"), length (rest)=w514) -> (substring=w509:string)
                n302 = String Subset(string=w516, offset (0)=0 ("偏移量(0)"), length (rest)=w515) -> (substring=w511:string)
                n303 = String Subset(string=w516, offset (0)=w515, length (rest)=w514) -> (substring=w510:string)
              }
              frame #1 {
                w525 = "\\"
                n304 = Concatenate Strings(w529, w528, w525, w527, w525, w526, w525) -> (w523:string)
                n305 = Concatenate Strings(w523, w522, w521) -> (w520:string)
                n306 = String To Path(string=w523) -> (path=w524:path)
                n307 = String To Path(string=w520) -> (path=w519:path)
              }
              frame #2 {
                n308 = call <vilib>:"Check if File or Folder Exists.vi"("path"=w531) -> ("file or folder exists?"=w532:bool)  [unwired: 8 in, 2 out]
                n309 = case shown="假" w532 {
                  tunnel: w531 -> [w533 _]
                  frame False {
                    n310 = Create Folder "创建文件夹"(path (use dialog)=w533) -> ()  [unwired: 2 in, 3 out]
                  }
                  frame True {
                  }
                }
              }
              frame #3 {
                n311 = control-ref of="本VI"() -> (w536:refnum<vi>)
                n312 = invoke class="VI" method="FP.Get Image"(reference=w536) -> ("image data"=w534:T1)  [unwired: 5 in, 5 out]
                n313 = call <vilib>:"Write JPEG File.vi"("image data"=w534, "path to JPEG file"=w535) -> ()  [unwired: 8 in, 2 out]
              }
            }
          }
          frame #2 {
            n314 = local write "流水线工步号"(660.0 ("工步号")) -> ()
          }
        }
      }
      frame 601 {
        n315 = flat-sequence {
          frame #0 {
            n316 = Wait (ms)(milliseconds to wait=u32 500 ("等待时间（毫秒）")) -> ()  [unwired: 1 out]
            n317 = flat-sequence {
              tunnel: ["F:\\报表存储\\"] -> w546
              tunnel: [w553] -> w545
              tunnel: [w552] -> w544
              tunnel: [w551] -> w543
              tunnel: [w548] -> w542
              tunnel: [".JPG"] -> w541
              tunnel: w546 -> [w571]
              tunnel: w545 -> [w570]
              tunnel: w544 -> [w569]
              tunnel: w543 -> [w568]
              tunnel: [w566] -> w540
              tunnel: w542 -> [w564]
              tunnel: w541 -> [w563]
              tunnel: [w561] -> w539
              tunnel: w540 -> [w573]
              tunnel: w539 -> [w572]
              tunnel: [w572] -> w538
              tunnel: w538 -> [w577]
              frame #0 {
                w556 = 2 ("长度（剩余）")
                w557 = 4 ("长度（剩余）")
                n318 = local read "产品ID"() -> (w550:string)
                n319 = Format Date/Time String(time format string (%c)="%Y%m%d") -> (date/time string=w558:string)  [unwired: 2 in]
                n320 = call <vilib>:"Trim Whitespace.vi"("string"=w550) -> ("trimmed string"=w548:string)  [unwired: 1 in]
                n321 = String Subset(string=w558, offset (0)=6 ("长度（剩余）"), length (rest)=w556) -> (substring=w551:string)
                n322 = String Subset(string=w558, offset (0)=0 ("偏移量(0)"), length (rest)=w557) -> (substring=w553:string)
                n323 = String Subset(string=w558, offset (0)=w557, length (rest)=w556) -> (substring=w552:string)
              }
              frame #1 {
                w567 = "\\"
                n324 = Concatenate Strings(w571, w570, w567, w569, w567, w568, w567) -> (w565:string)
                n325 = Concatenate Strings(w565, w564, w563) -> (w562:string)
                n326 = String To Path(string=w565) -> (path=w566:path)
                n327 = String To Path(string=w562) -> (path=w561:path)
              }
              frame #2 {
                n328 = call <vilib>:"Check if File or Folder Exists.vi"("path"=w573) -> ("file or folder exists?"=w574:bool)  [unwired: 8 in, 2 out]
                n329 = case shown="假" w574 {
                  tunnel: w573 -> [w575 _]
                  frame False {
                    n330 = Create Folder(path (use dialog)=w575) -> ()  [unwired: 2 in, 3 out]
                  }
                  frame True {
                  }
                }
              }
              frame #3 {
                n331 = control-ref of="本VI"() -> (w578:refnum<vi>)
                n332 = invoke class="VI" method="FP.Get Image"(reference=w578) -> ("image data"=w576:T1)  [unwired: 5 in, 5 out]
                n333 = call <vilib>:"Write JPEG File.vi"("image data"=w576, "path to JPEG file"=w577) -> ()  [unwired: 8 in, 2 out]
              }
            }
          }
          frame #1 {
            n334 = local write "流水线工步号"(660.0 ("工步号")) -> ()
          }
        }
      }
    }
    n335 = Wait Until Next ms Multiple(millisecond multiple=u32 50 ("毫秒倍数")) -> ()  [unwired: 1 out]
    n336 = local read "停止"() -> (w455:bool)
  }
  n337 = while {
    stop <- w580 stop-if-true
    n338 = event shown="[2] \"参数保存\": 值改变" {
      selector: _ -> [_ _ _ _ _ _]
      dyn-events: _ -> [_ _ _ _ _ _]
      timeout: 500 -> [_ _ _ _ _ _]
      event Timeout {
        n339 = event-data() -> ()  [unwired: 3 out]
      }
      event "参数查询": Value Change {
        n340 = event-data() -> ()  [unwired: 7 out]
        n341 = flat-sequence {
          tunnel: [w592] -> w588
          tunnel: [w601] -> w587
          tunnel: [w598] -> w586
          tunnel: [w595] -> w585
          tunnel: w588 -> [w606]
          tunnel: w587 -> [w604]
          tunnel: [w605] -> w584
          tunnel: w586 -> [w605]
          tunnel: [w604] -> w583
          tunnel: w585 -> [w603]
          tunnel: w584 -> [w609]
          tunnel: w583 -> [w608]
          frame #0 {
            n342 = call "字符串转换为数组.vi"("查询内容"=",产品型号,输入轴电机快进位置,输入轴电机快进速度,输入轴电机回零位置,输入轴电机慢进位置2,输入轴电机慢进位置3,输入轴电机慢进速度,输入轴电机测试位置,旋转电机位置1,旋转电机位置2,旋转电机速度,换向扭矩,检测扭矩,间隙合格判定值") -> ("列首"=w589:string[])  [unwired: 10 in]
            n343 = property on="参数列表" class="Tbl (严格)"("Row Headers[]"=w589) -> ()  [unwired: 2 in, 2 out]
          }
          frame #1 {
            n344 = call "ADO Connection Create.vi"() -> ("error out"=w597:errorcluster, "ADODB._Connection Out"=w600:refnum<k7>)  [unwired: 10 in]
            n345 = call "创建文本"() -> ("Result"=w602:string)  [unwired: 14 in, 1 out]
            n346 = call "ADO Connection Open.vi"("error in (no error)"=w597, "ConnectionString"="DSN=参数Z040;", "ADODB._Connection In"=w600) -> ("error out"=w596:errorcluster, "ADODB._Connection Out"=w591:refnum<k7>)  [unwired: 7 in]
            n347 = call "SQL Execute.vi"("error in (no error)"=w596, "Command Text"=w602, "ADODB._Connection In"=w591) -> ("error out"=w601:errorcluster, "Data"=w594:string[][], "ADODB._Connection Out"=w598:refnum<k7>)  [unwired: 5 in, 1 out]
            n348 = Transpose 2D Array "二维数组转置"(2D array=w594) -> (transposed array=w592:string[][])
            n349 = Index Array(array=w592, index (row)=0 ("索引 (行)")) -> (element=w595:string[])  [unwired: 1 in]
          }
          frame #2 {
            n350 = property on="参数列表" class="Tbl (严格)"("Column Headers[]"=w603) -> ()  [unwired: 2 in, 2 out]
            n351 = local write "参数列表"(w606) -> ()
          }
          frame #3 {
            n352 = call "ADO Connection Close.vi"("error in (no error)"=w608, "ADODB._Connection In"=w609) -> ("error out"=→"error out":errorcluster)  [unwired: 8 in, 1 out]
          }
        }
      }
      event "参数保存": Value Change {
        n353 = event-data() -> ()  [unwired: 7 out]
        n354 = while {
          i -> [w645]
          stop <- w648 stop-if-true
          n355 = local read "型号数量"() -> (w647:dbl)
          n356 = Greater Or Equal?(x=w645, y=w647) -> (x >= y?=w648:bool)
          n357 = Wait Until Next ms Multiple(millisecond multiple=u32 50 ("毫秒倍数")) -> ()  [unwired: 1 out]
          n358 = Index Array(array="参数列表", index (col)=w645) -> (element=w644:string[])  [unwired: 1 in]
          n359 = Index Array(array=w644, index #1=0, index #2=1, index #3=2, index #4=3, index #5=4, index #6=5, index #7=6, index #8=7, index #9=8, index #10=9, index #11=10, index #12=11, index #13=12, index #14=13) -> (element #1=w617:string, element #2=w630:string, element #3=w629:string, element #4=w628:string, element #5=w627:string, element #6=w626:string, element #7=w625:string, element #8=w624:string, element #9=w623:string, element #10=w622:string, element #11=w621:string, element #12=w620:string, element #13=w619:string, element #14=w618:string)
          n360 = call "创建文本4"("输入轴电机快进位置"=w630, "输入轴电机快进速度"=w629, "输入轴电机初始位置"=w628, "输入轴电机慢进位置2"=w627, "输入轴电机慢进位置3"=w626, "输入轴电机慢进速度"=w625, "输入轴电机最终位置"=w624, "旋转电机位置1"=w623, "旋转电机位置2"=w622, "旋转电机速度"=w621, "换向扭矩"=w620, "检测扭矩"=w619, "间隙合格判定值"=w618, "产品型号"=w617) -> ("Result"=w614:string)  [unwired: 12 in, 1 out]
          n361 = local read "ADODB._Connection Out"() -> (w610:refnum<k7>)
          n362 = call "SQL Execute.vi"("Command Text"=w614, "ADODB._Connection In"=w610) -> ("error out"=w616:errorcluster, "ADODB._Connection Out"=w615:refnum<k7>)  [unwired: 6 in, 2 out]
          n363 = call "ADO Connection Close.vi"("error in (no error)"=w616, "ADODB._Connection In"=w615) -> ("error out"=→"error out 5":errorcluster)  [unwired: 8 in, 1 out]
        }
      }
      event "传感器参数保存": Value Change {
        n364 = event-data() -> ()  [unwired: 7 out]
        n365 = local read "位移传感器比例偏移"() -> (w649:dbl)
        n366 = local read "位移传感器零点偏移"() -> (w650:dbl)
        n367 = local read "扭矩传感器比例偏移"() -> (w651:dbl)
        n368 = local read "扭矩传感器零点偏移"() -> (w652:dbl)
        n369 = Number To Fractional String(number=w650, precision (6)=i16 1 ("精度(6)")) -> (F-format string=w656:string)  [unwired: 2 in]
        n370 = Number To Fractional String(number=w651, precision (6)=i16 2 ("精度(6)")) -> (F-format string=w657:string)  [unwired: 2 in]
        n371 = Number To Fractional String(number=w652, precision (6)=i16 3 ("精度(6)")) -> (F-format string=w658:string)  [unwired: 2 in]
        n372 = Number To Fractional String(number=w649, precision (6)=i16 2 ("精度(6)")) -> (F-format string=w655:string)  [unwired: 2 in]
        n373 = call "创建文本2"("位移1比例偏移值"=w655, "压力1零点偏移值"=w658, "压力1比例偏移值"=w657, "位移1零点偏移值"=w656) -> ("Result"=w654:string)  [unwired: 10 in, 1 out]
        n374 = call "ADO Connection Create.vi"() -> ("error out"=w665:errorcluster, "ADODB._Connection Out"=w667:refnum<k7>)  [unwired: 10 in]
        n375 = call "ADO Connection Open.vi"("error in (no error)"=w665, "ConnectionString"="DSN=参数Z040;", "ADODB._Connection In"=w667) -> ("error out"=w664:errorcluster, "ADODB._Connection Out"=w666:refnum<k7>)  [unwired: 7 in]
        n376 = call "SQL Execute.vi"("error in (no error)"=w664, "Command Text"=w654, "ADODB._Connection In"=w666) -> ("error out"=w668:errorcluster, "ADODB._Connection Out"=w669:refnum<k7>)  [unwired: 5 in, 2 out]
        n377 = call "ADO Connection Close.vi"("error in (no error)"=w668, "ADODB._Connection In"=w669) -> ("error out"=→"error out 3":errorcluster)  [unwired: 8 in, 1 out]
      }
      event "停止": Value Change {
        n378 = event-data() -> ()  [unwired: 7 out]
        n379 = flat-sequence {
          frame #0 {
            n380 = local write "流水线工步号"(0.0 ("工步号")) -> ()
          }
          frame #1 {
            n381 = Wait Until Next ms Multiple(millisecond multiple=u32 1000 ("毫秒倍数")) -> ()  [unwired: 1 out]
          }
          frame #2 {
            n382 = Quit LabVIEW(quit? (T)=TRUE ("停止？(T)")) -> ()
          }
        }
      }
      event "电机回零": Mouse Down {
        n383 = event-data() -> ()  [unwired: 9 out]
        n384 = flat-sequence {
          tunnel: [w681] -> w677
          tunnel: w677 -> [w684]
          tunnel: [w684] -> w676
          tunnel: w676 -> [w686]
          tunnel: [w686] -> w675
          tunnel: w675 -> [w687]
          tunnel: [w687] -> w674
          tunnel: [w688] -> w679
          tunnel: w674 -> [w689]
          tunnel: w679 -> [w694]
          tunnel: [w694] -> w678
          tunnel: w678 -> [w696]
          tunnel: [w696] -> w680
          tunnel: [w695] -> w673
          tunnel: w680 -> [w707]
          tunnel: w673 -> [w706]
          frame #0 {
            n385 = local read "输入轴AxisHandle OUT"() -> (w681:u32)
            n386 = call "PCI1220U使能.vi"("使能"=TRUE, "AxisHandle IN"=w681) -> ()  [unwired: 9 in, 1 out]
          }
          frame #1 {
            n387 = Wait Until Next ms Multiple(millisecond multiple=u32 50 ("毫秒倍数")) -> ()  [unwired: 1 out]
          }
          frame #2 {
            n388 = local write "进给速度"(10.0 ("进给速度")) -> ()
          }
          frame #3 {
          }
          frame #4 {
            n389 = call <userlib>:"Acm_AxHome.vi"("DirMode"=u32 1, "HomeMode"=u32 11, "AxisHandle"=w689) -> ("ReturnValue"=→"ReturnValue":u32, "AxisHandle"=w688:u32)  [unwired: 1 in, 1 out]
          }
          frame #5 {
            n390 = Wait (ms)(milliseconds to wait=u32 100 ("等待时间（毫秒）")) -> ()  [unwired: 1 out]
          }
          frame #6 {
            n391 = while {
              tunnel: w696 -> [w705]
              tunnel: [w697] -> w695
              stop <- w698 stop-if-true
              n392 = local read "急停按钮"() -> (w702:bool)
              n393 = local read "复位按钮"() -> (w699:bool)
              n394 = call <userlib>:"Acm_AxGetCmdVelocity.vi"("AxisHandle"=w705) -> ("Velocity"=w704:dbl, "AxisHandle"=w697:u32)  [unwired: 1 in, 2 out]
              n395 = Equal To 0?(x=w704) -> (x = 0?=w701:bool)
              n396 = Not(x=w702) -> (.not. x?=w700:bool)
              n397 = Wait Until Next ms Multiple(millisecond multiple=u32 50 ("毫秒倍数")) -> ()  [unwired: 1 out]
              n398 = Compound Arithmetic op=OR(w701, w700, w699) -> (w698:bool)
            }
          }
          frame #7 {
            n399 = call "PCI1220U角度置零.vi"("AxisHandle IN"=w707) -> ()  [unwired: 10 in, 1 out]
            n400 = call "PCI1220U停止.vi"("AxisHandle IN"=w706) -> ()  [unwired: 9 in, 2 out]
          }
          frame #8 {
            n401 = local write "电机回零"(FALSE ("回零")) -> ()
          }
        }
      }
    }
    n402 = local read "停止"() -> (w580:bool)
    n403 = Wait Until Next ms Multiple(millisecond multiple=u32 200 ("毫秒倍数")) -> ()  [unwired: 1 out]
  }
  n404 = while {
    stop <- w709 stop-if-true
    n405 = stacked-sequence {
      frame #0 {
        n406 = First Call?() -> (First Call?: T/F=w712:bool)
        n407 = case shown="真" w712 {
          frame False {
          }
          frame True {
            w713 = TRUE ("旋转伺服使能")
            n408 = call "员工管理测试程序.vi"() -> ("员工姓名"=w715:string, "员工ID"=→"员工ID":string)  [unwired: 10 in]
            n409 = local write "旋转伺服使能"(w713) -> ()
            n410 = local write "输入轴使能"(w713) -> ()
            n411 = local write "员工姓名"(w715) -> ()
          }
        }
        "阻挡 2" <- "阻挡"
      }
      frame #1 {
        n412 = local read "报警工步号"() -> (w717:dbl)
        n413 = local read "测试 工步号"() -> (w719:dbl)
        n414 = local read "流水线工步号"() -> (w724:dbl)
        n415 = case shown="548" w724 {
          tunnel: [w784 "首先取下装钢球的辅具，准备放钢球" ("工步操作状态") "判断上序是否合格" ("工步操作状态") "自动放钢球启动" ("工步操作状态") "读取RFID信号" ("工步操作状态") "放钢球结束" ("工步操作状态") "补钢球" ("工步操作状态") "上阻挡器放行" ("工步操作状态") "装钢球辅具放回" ("工步操作状态") "取拧紧辅具" ("工步操作状态") "本工位检测" ("工步操作状态") "流水线气缸顶升" ("工步操作状态") "左标准气缸前进 " ("工步操作状态") "右标准气缸前进" ("工步操作状态") "等待测试开始" ("工步操作状态") "拧紧辅具放回" ("工步操作状态") "等待伺服电机对花键" ("工步操作状态") "给出本工位完成信号" ("工步操作状态") "右标准气缸回退" ("工步操作状态") "取气动定扭扳手加力" ("工步操作状态") "请放回辅具" ("工步操作状态") "流水线顶升气缸下降" ("工步操作状态") "本工位放行" ("工步操作状态") "放行完成" ("工步操作状态") "流水线位动作完成" ("工步操作状态") "本序已做，请复位！！！" ("工步操作状态") "本工位放行" ("工步操作状态") "放行完成" ("工步操作状态") "补钢球完成" ("工步操作状态") "循环结束" ("工步操作状态")] -> w723
          frame 0, Default {
            n416 = local read "联线按钮"() -> (w783:bool)
            n417 = case shown="假" w783 {
              tunnel: ["等待工件" "等待扫描条码" ("工步操作状态")] -> w784
              frame False {
              }
              frame True {
              }
            }
          }
          frame 5 {
          }
          frame 10 {
          }
          frame 20 {
          }
          frame 30 {
          }
          frame 40 {
          }
          frame 60 {
          }
          frame 70 {
          }
          frame 80 {
          }
          frame 85 {
          }
          frame 90 {
          }
          frame 95 {
          }
          frame 100 {
          }
          frame 110 {
          }
          frame 120 {
          }
          frame 130 {
          }
          frame 140 {
          }
          frame 520 {
          }
          frame 530 {
          }
          frame 545 {
          }
          frame 548 {
          }
          frame 550 {
          }
          frame 560 {
          }
          frame 580 {
          }
          frame 660 {
          }
          frame 800 {
          }
          frame 705 {
          }
          frame 710 {
          }
          frame 810 {
          }
          frame 900 {
          }
        }
        "流水线操作状态" <- w723
        n418 = case shown="1" w717 {
          tunnel: ["无报警" ("工步操作状态") "急停按钮被按下" ("工步操作状态") "输入轴电机报警" ("工步操作状态") "旋转电机报警" ("工步操作状态") "放钢球" ("工步操作状态") "放钢球结束" ("工步操作状态") "补钢球" ("工步操作状态") "装钢球气缸下降" ("工步操作状态") "装钢球辅具放回" ("工步操作状态") "取拧紧辅具" ("工步操作状态") "自动拧紧启动" ("工步操作状态") "拧紧气缸下降 " ("工步操作状态") "拧紧机启动" ("工步操作状态") "拧紧气缸退回" ("工步操作状态") "拧紧辅具放回" ("工步操作状态") "测间隙启动" ("工步操作状态") "上测间隙下降" ("工步操作状态") "下测间隙上" ("工步操作状态") "下测间隙回" ("工步操作状态") "判断合格不合格" ("工步操作状态") "上测间隙回" ("工步操作状态") "压铆启动" ("工步操作状态") "增压缸快进" ("工步操作状态") "增压缸增压" ("工步操作状态") "压铆力判断" ("工步操作状态") "增压缸退回" ("工步操作状态") "不合格品，复位解除" ("工步操作状态") "补钢球完成" ("工步操作状态") "循环结束" ("工步操作状态")] -> w716
          frame 0, Default {
          }
          frame 1 {
          }
          frame 2 {
          }
          frame 4 {
          }
          frame 30 {
          }
          frame 40 {
          }
          frame 60 {
          }
          frame 70 {
          }
          frame 80 {
          }
          frame 85 {
          }
          frame 90 {
          }
          frame 100 {
          }
          frame 110 {
          }
          frame 120 {
          }
          frame 130 {
          }
          frame 140 {
          }
          frame 150 {
          }
          frame 160 {
          }
          frame 170 {
          }
          frame 175 {
          }
          frame 176 {
          }
          frame 180 {
          }
          frame 190 {
          }
          frame 200 {
          }
          frame 210 {
          }
          frame 211 {
          }
          frame 800 {
          }
          frame 810 {
          }
          frame 900 {
          }
        }
        "报警信息" <- w716
        n419 = case shown="120" w719 {
          tunnel: ["等待流水线准备好信号" ("工步操作状态") "首先取下装钢球的辅具，准备放钢球" ("工步操作状态") "装钢球气缸顶起" ("工步操作状态") "输入轴伺服电机下降，旋转伺服左右旋转对取花键" ("工步操作状态") "放钢球" ("工步操作状态") "标准气缸左前进" ("工步操作状态") "右标准气缸前进" ("工步操作状态") "装钢球气缸下降" ("工步操作状态") "导杆气缸前进" ("工步操作状态") "取拧紧辅具" ("工步操作状态") "自动拧紧启动" ("工步操作状态") "等待输入轴电机初始位置完成 " ("工步操作状态") "导杆气缸下降" ("工步操作状态") "间隙测试开始" ("工步操作状态") "导杆气缸回退" ("工步操作状态") "测间隙测试结束" ("工步操作状态") "上测间隙下降" ("工步操作状态") "下测间隙上" ("工步操作状态") "下测间隙回" ("工步操作状态") "判断合格不合格" ("工步操作状态") "上测间隙回" ("工步操作状态") "压铆启动" ("工步操作状态") "增压缸快进" ("工步操作状态") "增压缸增压" ("工步操作状态") "压铆力判断" ("工步操作状态") "增压缸退回" ("工步操作状态") "不合格品，复位解除" ("工步操作状态") "补钢球完成" ("工步操作状态") "循环结束" ("工步操作状态")] -> w718
          frame 0, Default {
          }
          frame 5 {
          }
          frame 10 {
          }
          frame 20 {
          }
          frame 30 {
          }
          frame 40 {
          }
          frame 60 {
          }
          frame 70 {
          }
          frame 80 {
          }
          frame 85 {
          }
          frame 90 {
          }
          frame 100 {
          }
          frame 110 {
          }
          frame 120 {
          }
          frame 130 {
          }
          frame 140 {
          }
          frame 150 {
          }
          frame 160 {
          }
          frame 170 {
          }
          frame 175 {
          }
          frame 176 {
          }
          frame 180 {
          }
          frame 190 {
          }
          frame 200 {
          }
          frame 210 {
          }
          frame 211 {
          }
          frame 800 {
          }
          frame 810 {
          }
          frame 990 {
          }
        }
        "测试操作状态" <- w718
        n420 = local read "输入轴AxisHandle OUT"() -> (w720:u32)
        n421 = call <userlib>:"Acm_AxDiGetBit.vi"("DiChannel"=u16 3, "AxisHandle"=w720) -> ("ReturnValue"=→"ReturnValue 3":u32)  [unwired: 2 in, 3 out]
      }
      frame #2 {
        n422 = local read "力矩（nm)"() -> (w821:dbl)
        n423 = local read "电机下降"() -> (w823:bool)
        n424 = local read "电机上升"() -> (w822:bool)
        n425 = Absolute Value(x=w821) -> (abs(x)=w820:dbl)
        n426 = Not(x=w822) -> (.not. x?=w818:bool)
        n427 = Less?(x=w820, y=20.0) -> (x < y?=w817:bool)
        n428 = Compound Arithmetic op=AND(w823, w818, w817) -> (w816:bool)
        n429 = case shown="真" w816 {
          frame False {
          }
          frame True {
            n430 = flat-sequence {
              tunnel: [w829] -> w825
              tunnel: w825 -> [w832]
              tunnel: [w832] -> w824
              tunnel: w824 -> [w833]
              tunnel: [w833] -> w826
              tunnel: w826 -> [w845]
              frame #0 {
                n431 = local write "输入轴使能"(TRUE ("输入轴使能")) -> ()
              }
              frame #1 {
                n432 = local write "进给速度"(5.0 ("进给速度")) -> ()
              }
              frame #2 {
                n433 = local read "输入轴AxisHandle OUT"() -> (w831:u32)
                n434 = call "PCI1220U运行.vi"("方向"=u16 0, "AxisHandle IN"=w831) -> ("AxisHandle OUT"=w829:u32)  [unwired: 9 in]
              }
              frame #3 {
              }
              frame #4 {
                n435 = while {
                  stop <- w837 stop-if-true
                  n436 = local read "力矩（nm)"() -> (w840:dbl)
                  n437 = local read "急停按钮"() -> (w836:bool)
                  n438 = local read "复位按钮"() -> (w834:bool)
                  n439 = local read "电机下降"() -> (w844:bool)
                  n440 = Absolute Value(x=w840) -> (abs(x)=w841:dbl)
                  n441 = Greater Or Equal?(x=w841, y=20.0) -> (x >= y?=w838:bool)
                  n442 = Not(x=w836) -> (.not. x?=w835:bool)
                  n443 = Not(x=w844) -> (.not. x?=w839:bool)
                  n444 = Wait Until Next ms Multiple(millisecond multiple=u32 50 ("毫秒倍数")) -> ()  [unwired: 1 out]
                  n445 = Compound Arithmetic op=OR(w839, w838, w835, w834) -> (w837:bool)
                }
              }
              frame #5 {
                n446 = call "PCI1220U停止.vi"("AxisHandle IN"=w845) -> ()  [unwired: 9 in, 2 out]
              }
            }
          }
        }
      }
      frame #3 {
        n447 = local read "力矩（nm)"() -> (w853:dbl)
        n448 = local read "电机上升"() -> (w847:bool)
        n449 = local read "电机下降"() -> (w846:bool)
        n450 = Absolute Value(x=w853) -> (abs(x)=w852:dbl)
        n451 = Not(x=w846) -> (.not. x?=w850:bool)
        n452 = Less?(x=w852, y=20.0) -> (x < y?=w849:bool)
        n453 = Compound Arithmetic op=AND(w847, w850, w849) -> (w848:bool)
        n454 = case shown="真" w848 {
          frame False {
          }
          frame True {
            n455 = flat-sequence {
              tunnel: [w859] -> w856
              tunnel: w856 -> [w862]
              tunnel: [w862] -> w855
              tunnel: w855 -> [w863]
              tunnel: [w863] -> w854
              tunnel: w854 -> [w876]
              frame #0 {
                n456 = local write "输入轴使能"(TRUE ("输入轴使能")) -> ()
              }
              frame #1 {
                n457 = local write "进给速度"(5.0 ("进给速度")) -> ()
              }
              frame #2 {
                n458 = local read "输入轴AxisHandle OUT"() -> (w861:u32)
                n459 = call "PCI1220U运行.vi"("方向"=u16 1, "AxisHandle IN"=w861) -> ("AxisHandle OUT"=w859:u32)  [unwired: 9 in]
              }
              frame #3 {
              }
              frame #4 {
                n460 = while {
                  stop <- w872 stop-if-true
                  n461 = local read "力矩（nm)"() -> (w868:dbl)
                  n462 = local read "电机上升"() -> (w871:bool)
                  n463 = local read "急停按钮"() -> (w866:bool)
                  n464 = local read "复位按钮"() -> (w864:bool)
                  n465 = Absolute Value(x=w868) -> (abs(x)=w869:dbl)
                  n466 = Not(x=w871) -> (.not. x?=w873:bool)
                  n467 = Greater Or Equal?(x=w869, y=20.0) -> (x >= y?=w867:bool)
                  n468 = Not(x=w866) -> (.not. x?=w865:bool)
                  n469 = Wait Until Next ms Multiple(millisecond multiple=u32 50 ("毫秒倍数")) -> ()  [unwired: 1 out]
                  n470 = Compound Arithmetic op=OR(w873, w867, w865, w864) -> (w872:bool)
                }
              }
              frame #5 {
                n471 = call "PCI1220U停止.vi"("AxisHandle IN"=w876) -> ()  [unwired: 9 in, 2 out]
                n472 = Wait (ms)(milliseconds to wait=u32 100 ("毫秒计时值")) -> ()  [unwired: 1 out]
              }
            }
          }
        }
      }
      frame #4 {
        n473 = local read "右旋"() -> (w877:bool)
        n474 = local read "力矩（nm)"() -> (w884:dbl)
        n475 = local read "左旋"() -> (w878:bool)
        n476 = Absolute Value(x=w884) -> (abs(x)=w883:dbl)
        n477 = Not(x=w877) -> (.not. x?=w881:bool)
        n478 = Less?(x=w883, y=20.0) -> (x < y?=w880:bool)
        n479 = Compound Arithmetic op=AND(w878, w881, w880) -> (w879:bool)
        n480 = case shown="真" w879 {
          frame False {
          }
          frame True {
            n481 = flat-sequence {
              tunnel: [w891] -> w885
              tunnel: [w892] -> w886
              tunnel: w885 -> [w892]
              tunnel: [w895] -> w889
              tunnel: w886 -> [w894]
              tunnel: w889 -> [w897]
              tunnel: [w897] -> w888
              tunnel: w888 -> [w898]
              tunnel: [w898] -> w887
              tunnel: w887 -> [w911]
              frame #0 {
                n482 = local read "旋转轴AxisHandle OUT"() -> (w891:u32)
                n483 = local write "旋转伺服使能"(TRUE ("旋转伺服使能")) -> ()
              }
              frame #1 {
                n484 = local write "旋转速度"(10.0 ("进给速度")) -> ()
              }
              frame #2 {
                n485 = call "PCI1220U运行.vi"("方向"=u16 0, "AxisHandle IN"=w894) -> ("AxisHandle OUT"=w895:u32)  [unwired: 9 in]
              }
              frame #3 {
              }
              frame #4 {
                n486 = while {
                  stop <- w907 stop-if-true
                  n487 = local read "力矩（nm)"() -> (w904:dbl)
                  n488 = local read "急停按钮"() -> (w902:bool)
                  n489 = local read "左旋"() -> (w899:bool)
                  n490 = local read "复位按钮"() -> (w900:bool)
                  n491 = Absolute Value(x=w904) -> (abs(x)=w905:dbl)
                  n492 = Not(x=w899) -> (.not. x?=w908:bool)
                  n493 = Greater Or Equal?(x=w905, y=20.0) -> (x >= y?=w903:bool)
                  n494 = Not(x=w902) -> (.not. x?=w901:bool)
                  n495 = Wait Until Next ms Multiple(millisecond multiple=u32 50 ("毫秒倍数")) -> ()  [unwired: 1 out]
                  n496 = Compound Arithmetic op=OR(w908, w903, w901, w900) -> (w907:bool)
                }
              }
              frame #5 {
                n497 = call "PCI1220U停止.vi"("AxisHandle IN"=w911) -> ()  [unwired: 9 in, 2 out]
                n498 = Wait (ms)(milliseconds to wait=u32 100 ("毫秒计时值")) -> ()  [unwired: 1 out]
              }
            }
          }
        }
      }
      frame #5 {
        n499 = local read "力矩（nm)"() -> (w919:dbl)
        n500 = local read "右旋"() -> (w913:bool)
        n501 = local read "左旋"() -> (w912:bool)
        n502 = Absolute Value(x=w919) -> (abs(x)=w918:dbl)
        n503 = Not(x=w912) -> (.not. x?=w916:bool)
        n504 = Less?(x=w918, y=20.0) -> (x < y?=w915:bool)
        n505 = Compound Arithmetic op=AND(w913, w916, w915) -> (w914:bool)
        n506 = case shown="真" w914 {
          frame False {
          }
          frame True {
            n507 = flat-sequence {
              tunnel: [w926] -> w920
              tunnel: [w928] -> w921
              tunnel: w920 -> [w928]
              tunnel: [w930] -> w924
              tunnel: w921 -> [w929]
              tunnel: w924 -> [w932]
              tunnel: [w932] -> w923
              tunnel: w923 -> [w933]
              tunnel: [w933] -> w922
              tunnel: w922 -> [w946]
              frame #0 {
                n508 = local read "旋转轴AxisHandle OUT"() -> (w926:u32)
                n509 = local write "旋转伺服使能"(TRUE ("旋转伺服使能")) -> ()
              }
              frame #1 {
                n510 = local write "旋转速度"(10.0 ("进给速度")) -> ()
              }
              frame #2 {
                n511 = call "PCI1220U运行.vi"("方向"=u16 1, "AxisHandle IN"=w929) -> ("AxisHandle OUT"=w930:u32)  [unwired: 9 in]
              }
              frame #3 {
              }
              frame #4 {
                n512 = while {
                  stop <- w942 stop-if-true
                  n513 = local read "力矩（nm)"() -> (w939:dbl)
                  n514 = local read "右旋"() -> (w934:bool)
                  n515 = local read "急停按钮"() -> (w937:bool)
                  n516 = local read "复位按钮"() -> (w935:bool)
                  n517 = Absolute Value(x=w939) -> (abs(x)=w940:dbl)
                  n518 = Not(x=w934) -> (.not. x?=w943:bool)
                  n519 = Greater Or Equal?(x=w940, y=20.0) -> (x >= y?=w938:bool)
                  n520 = Not(x=w937) -> (.not. x?=w936:bool)
                  n521 = Wait Until Next ms Multiple(millisecond multiple=u32 50 ("毫秒倍数")) -> ()  [unwired: 1 out]
                  n522 = Compound Arithmetic op=OR(w943, w938, w936, w935) -> (w942:bool)
                }
              }
              frame #5 {
                n523 = call "PCI1220U停止.vi"("AxisHandle IN"=w946) -> ()  [unwired: 9 in, 2 out]
                n524 = Wait (ms)(milliseconds to wait=u32 100 ("毫秒计时值")) -> ()  [unwired: 1 out]
              }
            }
          }
        }
      }
    }
    n525 = Wait Until Next ms Multiple(millisecond multiple=u32 50 ("毫秒倍数")) -> ()  [unwired: 1 out]
    n526 = local read "停止"() -> (w709:bool)
  }
  n527 = flat-sequence {
    tunnel: [w948] -> w6
    tunnel: [w947] -> w5
    tunnel: w6 -> [w955]
    tunnel: w5 -> [w954]
    tunnel: [w953] -> w4
    tunnel: [w952] -> w3
    tunnel: w4 -> [w1054]
    tunnel: w3 -> [w1053]
    frame #0 {
      n528 = call "ADO Connection Create.vi"() -> ("error out"=w950:errorcluster, "ADODB._Connection Out"=w951:refnum<k7>)  [unwired: 10 in]
      n529 = call "ADO Connection Open.vi"("error in (no error)"=w950, "ConnectionString"="DSN=参数Z040;", "ADODB._Connection In"=w951) -> ("error out"=w947:errorcluster, "ADODB._Connection Out"=w948:refnum<k7>)  [unwired: 7 in]
      "ADODB._Connection Out" <- w948
    }
    frame #1 {
      n530 = while {
        tunnel: w955 -> [w960]
        tunnel: w954 -> [w959]
        tunnel: [w958] -> w953
        tunnel: [w957] -> w952
        stop <- w963 stop-if-true
        n531 = local read "参数加载"() -> (w956:bool)
        n532 = Wait (ms)(milliseconds to wait=u32 200 ("等待时间（毫秒）")) -> ()  [unwired: 1 out]
        n533 = First Call?() -> (First Call?: T/F=w962:bool)
        n534 = Or(x=w962, y=w956) -> (x .or. y?=w961:bool)
        n535 = case shown="真" w961 {
          tunnel: w960 -> [w966 w970]
          tunnel: w959 -> [w965 w969]
          tunnel: [w966 w968] -> w958
          tunnel: [w965 w967] -> w957
          frame False {
          }
          frame True {
            n536 = stacked-sequence {
              seq-local: [w974 _ _] -> [_ w1037 _]
              tunnel: w970 -> [w975 w1034 _]
              tunnel: w969 -> [w976 _ _]
              tunnel: [w975 _ _] -> w968
              tunnel: [_ w1036 _] -> w967
              frame #0 {
                n537 = First Call?() -> (First Call?: T/F=w973:bool)
                n538 = local read "参数加载"() -> (w972:bool)
                n539 = Or(x=w973, y=w972) -> (x .or. y?=w971:bool)
                n540 = case shown="真" w971 {
                  tunnel: w976 -> [w977 w983]
                  tunnel: w975 -> [_ w981]
                  tunnel: [w977 w980] -> w974
                  frame False {
                  }
                  frame True {
                    n541 = call "SQL Execute.vi"("error in (no error)"=w983, "Command Text"="SELECT * FROM 测试参数表 ;", "ADODB._Connection In"=w981) -> ("error out"=w980:errorcluster, "Data"=w984:string[][])  [unwired: 5 in, 2 out]
                    n542 = Index Array "索引数组"(array=w984, index (col)=0 ("禁用的索引 (列)")) -> (element=w986:string[])  [unwired: 1 in]
                    n543 = Array Size "数组大小"(array=w986) -> (size(s)=w978:i32)
                    "型号数量" <- w978
                    n544 = while {
                      shift-right: [w991] -> w985
                      shift-left: i32[] [] -> [w992]
                      tunnel: w978 -> [w989]
                      i -> [w990]
                      stop <- w993 stop-if-true
                      n545 = Greater Or Equal?(x=w990, y=w989) -> (x >= y?=w993:bool)
                      n546 = Build Array (concatenate) "创建数组"(w992, w990) -> (w991:i32[])
                    }
                    n547 = Build Cluster Array "索引与捆绑簇数组"(w986, w985) -> (w979:cluster{"String":string, i32}[])
                    n548 = property on="型号选择" class="Ring (严格)"("StringsAndValues[]"=w979) -> ()  [unwired: 2 in, 2 out]
                  }
                }
              }
              frame #1 {
                (unwired) ",产品型号,输入轴电机快进位置,输入轴电机快进速度,输入轴电机慢进位置,输入轴电机慢进速度,旋转电机位置1,旋转电机位置2,旋转电机速度,换向扭矩,间隙判定值" ("查询内容")
                n549 = property on="型号选择" class="Ring (严格)"() -> ("RingText.Text"=w1033:string)  [unwired: 2 in, 2 out]
                n550 = call "创建文本3"("产品型号"=w1033) -> ("Result"=w1035:string)  [unwired: 13 in, 1 out]
                n551 = call "SQL Execute.vi"("error in (no error)"=w1037, "Command Text"=w1035, "ADODB._Connection In"=w1034) -> ("error out"=w1036:errorcluster, "Data"=w1039:string[][])  [unwired: 5 in, 2 out]
                n552 = Index Array "索引数组"(array=w1039, index (row)=0 ("索引 (行)")) -> (element=w1032:string[])  [unwired: 1 in]
                n553 = Fract/Exp String To Number "分数/指数字符串至数值转换"(string=w1032) -> (number=w1006:dbl[])  [unwired: 3 in, 1 out]
                n554 = Index Array(array=w1006, index #1=1 ("索引"), index #2=2 ("索引"), index #3=3 ("索引"), index #4=4 ("索引"), index #5=5 ("索引"), index #6=6 ("索引"), index #7=7 ("索引"), index #8=8 ("索引"), index #9=9 ("索引"), index #10=10 ("索引"), index #11=11 ("索引"), index #12=12 ("索引"), index #13=13 ("索引"), index #14=14 ("索引"), index #15=15 ("索引"), index #16=16 ("索引"), index #17=17 ("索引"), index #18=18 ("索引"), index #19=19 ("索引"), index #20=20 ("索引"), index #21=21 ("索引"), index #22=22 ("索引"), index #23=23 ("索引"), index #24=24 ("索引")) -> (element #1=w1005:dbl, element #2=→"输入轴电机快进速度":dbl, element #3=w1004:dbl, element #4=→"输入轴电机慢进位置2":dbl, element #5=→"输入轴电机慢进位置3":dbl, element #6=→"输入轴电机慢进速度":dbl, element #7=→"输入轴最终位置（mm)":dbl, element #8=w999:dbl, element #9=w998:dbl, element #10=→"旋转电机速度":dbl, element #11=w996:dbl, element #12=w995:dbl, element #13=w994:dbl)  [unwired: 11 out]
                n555 = local write "间隙合格标准值(mm)"(w994) -> ()
                n556 = local write "输入轴快进位置(mm)"(w1005) -> ()
                n557 = local write "旋转左极限位(mm)"(w999) -> ()
                n558 = local write "旋转右极限位(mm)"(w998) -> ()
                n559 = local write "换向扭矩(NM)"(w996) -> ()
                n560 = local write "检测扭矩(NM)"(w995) -> ()
                n561 = local write "输入轴初始位置(mm)"(w1004) -> ()
              }
              frame #2 {
                n562 = local read "ADODB._Connection Out"() -> (w1047:refnum<k7>)
                n563 = call "SQL Execute.vi"("Command Text"="SELECT * FROM 传感器校验表 where ID='2'", "ADODB._Connection In"=w1047) -> ("Data"=w1052:string[][])  [unwired: 6 in, 3 out]
                n564 = Index Array "索引数组"(array=w1052) -> (element=w1051:string[])  [unwired: 2 in]
                n565 = Fract/Exp String To Number "分数/指数字符串至数值转换"(string=w1051) -> (number=w1050:dbl[])  [unwired: 3 in, 1 out]
                n566 = Index Array "索引数组"(array=w1050, index #1=1 ("索引"), index #2=2 ("索引"), index #3=3 ("索引"), index #4=4 ("索引")) -> (element #1=w1043:dbl, element #2=w1042:dbl, element #3=w1041:dbl, element #4=w1040:dbl)
                n567 = local write "扭矩传感器零点偏移"(w1043) -> ()
                n568 = local write "扭矩传感器比例偏移"(w1042) -> ()
                n569 = local write "位移传感器零点偏移"(w1041) -> ()
                n570 = local write "位移传感器比例偏移"(w1040) -> ()
              }
            }
          }
        }
        n571 = local read "停止"() -> (w963:bool)
      }
    }
    frame #2 {
      n572 = call "ADO Connection Close.vi"("error in (no error)"=w1053, "ADODB._Connection In"=w1054) -> ("error out"=→"error out 2":errorcluster)  [unwired: 8 in, 1 out]
    }
  }
  n573 = flat-sequence {
    tunnel: [w1059] -> w9
    tunnel: [w1057] -> w2
    tunnel: [w1056] -> w1
    tunnel: w9 -> [w1063]
    tunnel: [w1062] -> w8
    tunnel: w2 -> [w1061]
    tunnel: w1 -> [w1060]
    tunnel: w8 -> [w1143]
    tunnel: [w1143] -> w7
    tunnel: w7 -> [w1145]
    frame #0 {
      n574 = call "PCI1240U初始化.vi"() -> ("2电机"=w1056:u32, "1电机"=w1057:u32, "DeviceHandle"=→"DeviceHandle":u32)  [unwired: 6 in, 3 out]
      "输入轴AxisHandle OUT" <- w1056
      "旋转轴AxisHandle OUT" <- w1057
      n575 = call "PCI8622配置.vi"() -> ("DeviceID"=w1059:i32)  [unwired: 11 in]
    }
    frame #1 {
      n576 = while {
        tunnel: w1063 -> [w1110]
        tunnel: [w1110] -> w1062
        tunnel: w1061 -> [w1076]
        tunnel: w1060 -> [w1075]
        stop <- "停止" stop-if-true
        w1120 = 0  # nRetSizeWords
        w1121 = 2048  # nReadSizeWords
        # "hDevice"
        n577 = Wait Until Next ms Multiple(millisecond multiple=u32 50 ("毫秒倍数")) -> ()  [unwired: 1 out]
        n578 = Initialize Array(u16 0, 2048 ("dimension size")) -> (w1111:u16[])
        n579 = call "PCI1220U使能.vi"("使能"="旋转伺服使能", "AxisHandle IN"=w1076) -> ()  [unwired: 9 in, 1 out]
        n580 = call "PCI1220U使能.vi"("使能"="输入轴使能", "AxisHandle IN"=w1075) -> ()  [unwired: 9 in, 1 out]
        n581 = dll-call lib="PCI8622_32.dll" fn="PCI8622_ReadDeviceProAD_Npt" label="ReadDeviceProAD_Npt"("hDevice"=w1110, "ADBuffer[]"=w1111, "nReadSizeWords"=w1121, "nRetSizeWords"=w1120) -> ("ADBuffer[]"=w1114:u16[])  [unwired: 7 in, 2 out]
        n582 = Divide(x=w1114, y=65536.01) -> (x/y=w1115:dbl[])
        n583 = Multiply(x=w1115, y=20) -> (x*y=w1118:dbl[])
        n584 = call "PCI1220U速度设置.vi"("Change Velocity"="旋转速度", "AxisHandle IN"=w1076) -> ("AxisHandle OUT"=w1080:u32)  [unwired: 9 in]
        n585 = call "PCI1220电动缸速度设置.vi"("Change Velocity"="进给速度", "AxisHandle IN"=w1075) -> ("AxisHandle OUT"=w1079:u32)  [unwired: 8 in]
        n586 = Subtract(x=w1118, y=10) -> (x-y=w1106:dbl[])
        n587 = Decimate 1D Array "抽取一维数组"(w1106) -> (w1086:dbl[], w1085:dbl[])  [unwired: 6 out]
        n588 = call "PCI1220电动缸读取位置.vi"("AxisHandle IN"=w1079) -> ("位置"=→"输入轴伺服位置":dbl)  [unwired: 9 in, 1 out]
        n589 = Add Array Elements(numeric array=w1085) -> (sum=w1095:dbl)
        n590 = Add Array Elements(numeric array=w1086) -> (sum=w1108:dbl)
        n591 = Array Size(array=w1085) -> (size(s)=w1094:i32)
        n592 = Array Size(array=w1086) -> (size(s)=w1107:i32)
        n593 = Divide(x=w1095, y=w1094) -> (x/y=w1093:dbl)
        n594 = Divide(x=w1108, y=w1107) -> (x/y=w1104:dbl)
        n595 = call "PCI1220U读取位置.vi"("AxisHandle IN"=w1080) -> ("位置"=→"旋转轴伺服位置":dbl)  [unwired: 9 in, 1 out]
        n596 = local read "扭矩传感器零点偏移"() -> (w1097:dbl)
        n597 = local read "位移传感器比例偏移"() -> (w1087:dbl)
        n598 = Subtract(x=w1093, y=4.1894) -> (x-y=w1091:dbl)
        n599 = Subtract(x=w1104, y=-0.0) -> (x-y=w1103:dbl)
        n600 = Multiply(x=w1091, y=1.0) -> (x*y=w1089:dbl)
        n601 = Multiply(x=w1103, y=5.0) -> (x*y=w1101:dbl)
        n602 = local read "扭矩传感器比例偏移"() -> (w1096:dbl)
        n603 = Subtract(x=w1089, y=0.0) -> (x-y=w1072:dbl)
        n604 = Subtract(x=w1101, y=0.0) -> (x-y=w1100:dbl)
        n605 = Subtract(x=w1100, y=w1097) -> (x-y=w1099:dbl)
        n606 = Multiply(x=w1072, y=w1087) -> (x*y=w1071:dbl)
        n607 = Multiply(x=w1099, y=w1096) -> (x*y=→"力矩（nm)":dbl)
        n608 = Add(x=w1071, y=0.04) -> (x+y=w1069:dbl)
        n609 = call "滤波器"("Signal"=w1069) -> ("Filtered Signal"=→"位移(mm)":dynamicdata)  [unwired: 9 in, 1 out]
        n610 = Equal?(x="密码", y="jizhuan") -> (x = y?=w1066:bool)
        n611 = Compound Arithmetic op=AND("确定按钮", w1066) -> (w1064:bool)
        n612 = case shown="真" w1064 {
          frame False {
            w1123 = T2."Disabled and Grayed Out" ("禁用")
            n613 = property on="确定按钮 2" class="Bool"("DisabledEnum"=w1123) -> ()  [unwired: 2 in, 2 out]
            n614 = property on="确定按钮 3" class="Bool"("DisabledEnum"=w1123) -> ()  [unwired: 2 in, 2 out]
          }
          frame True {
            n615 = property on="确定按钮 2" class="Bool"("DisabledEnum"=T2."Enabled" ("禁用")) -> ()  [unwired: 2 in, 2 out]
            n616 = property on="确定按钮 3" class="Bool"("DisabledEnum"=T2."Enabled" ("禁用")) -> ()  [unwired: 2 in, 2 out]
            n617 = case shown="真" "确定按钮 2" {
              frame False {
              }
              frame True {
                n618 = property on="选项卡控件 2" class="TabCtl (严格)"() -> ("Pages"=w1136:refnum<vi>[])  [unwired: 2 in, 2 out]
                n619 = property on="参数保存" class="Bool (严格)"("DisabledEnum"=T2."Disabled and Grayed Out" ("禁用")) -> ()  [unwired: 2 in, 2 out]
                n620 = for {
                  N: 4 -> [_]
                  tunnel: w1136 -> [w1138] mode=indexing
                  i -> [w1139]
                  n621 = case shown="2" w1139 {
                    tunnel: w1138 -> [_ w1141]
                    frame 0, Default {
                    }
                    frame 2 {
                      n622 = property class="Page"(reference=w1141, "PageVis"=FALSE ("选项卡可见")) -> ()  [unwired: 1 in, 2 out]
                    }
                  }
                }
              }
            }
            n623 = case shown="真" "确定按钮 3" {
              frame False {
              }
              frame True {
                n624 = property on="选项卡控件 2" class="TabCtl (严格)"() -> ("Pages"=w1129:refnum<vi>[])  [unwired: 2 in, 2 out]
                n625 = property on="参数保存" class="Bool (严格)"("DisabledEnum"=T2."Enabled" ("禁用")) -> ()  [unwired: 2 in, 2 out]
                n626 = for {
                  N: 4 -> [_]
                  tunnel: w1129 -> [w1131] mode=indexing
                  i -> [w1132]
                  n627 = case shown="2" w1132 {
                    tunnel: w1131 -> [_ w1134]
                    frame 0, Default {
                    }
                    frame 2 {
                      n628 = property class="Page"(reference=w1134, "PageVis"=TRUE ("选项卡可见")) -> ()  [unwired: 1 in, 2 out]
                    }
                  }
                }
              }
            }
          }
        }
      }
    }
    frame #2 {
      n629 = dll-call lib="PCI8622_32.dll" fn="PCI8622_StopDeviceProAD" label="StopDeviceProAD"("hDevice"=w1143) -> ("hDevice"=w1144:i32)  [unwired: 4 in, 2 out]
      n630 = local read "DeviceHandle"() -> (w1142:u32)
      n631 = dll-call lib="PCI8622_32.dll" fn="PCI8622_ReleaseDeviceProAD" label="ReleaseDeviceProAD"("hDevice"=w1144) -> ()  [unwired: 5 in, 2 out]
      n632 = call <userlib>:"Acm_DevClose.vi"("DeviceHandle"=w1142) -> ()  [unwired: 1 in, 2 out]
    }
    frame #3 {
      n633 = dll-call lib="PCI8622_32.dll" fn="PCI8622_ReleaseDevice" label="ReleaseDevice"("hDevice"=w1145) -> ()  [unwired: 5 in, 2 out]
    }
  }
